vi "AnalogAcquisition.vi"() -> ()   [LabVIEW 2017]
uses:
  <vilib>/DAQmx/create/channels.llb/DAQmx Create Channel (AI-Voltage-Basic).vi
  <vilib>/DAQmx/read.llb/DAQmx Read (Analog 1D DBL NChan 1Samp).vi
  <vilib>/DAQmx/configure/timing.llb/DAQmx Timing (Sample Clock).vi
  <vilib>/DAQmx/create/channels.llb/DAQmx Create Channel (AI-Current-Basic).vi
panel:
  out "KnobDistance 1.4":dbl[](array[numeric])
  out "KnobDistance 2.4":dbl[](array[numeric])
  out "KnobDistance 2.3":dbl[](array[numeric])
  out "KnobDistance 2.2":dbl[](array[numeric])
  out "KnobDistance 2.1":dbl[](array[numeric])
  out "KnobDistance 1.3":dbl[](array[numeric])
  out "KnobDistance 1.2":dbl[](array[numeric])
  out "KnobDistance 1.1":dbl[](array[numeric])
  out "BufferWDWArray 2.3":T1
  out "BufferWDWArray 2.4":T1
  out "BufferWDWArray 2.1":T1
  out "BufferWDWArray 2.2":T1
  out "BufferWDWArray 1.3":T1
  out "BufferWDWArray 1.4":T1
  out "BufferWDWArray 1.1":T1
  out "BufferWDWArray 1.2":T1
  out "WDW Judge 2":bool
  out "WDW Judge":bool
  out "SamplingRate":i32
  in  "stop":bool
  out "WDW_Read 2":bool
  out "RL_Read 2":bool
  out "FL_Read 2":bool
  out "RR_Read 2":bool
  out "FR_Read 2":bool
  out "DL_Read 2":bool
  out "RL_Read 1":bool
  out "FL_Read 1":bool
  out "RR_Read 1":bool
  out "FR_Read 1":bool
  out "DL_Read 1":bool
  out "WDW_Read 1":bool
  out "Flash":bool
  out "BufferRLArray 2.3":T2
  out "BufferRLArray 2.4":T2
  out "BufferFLArray 2.3":T2
  out "BufferFLArray 2.4":T2
  out "BufferRRArray 2.3":T2
  out "BufferRRArray 2.4":T2
  out "BufferFRArray 2.3":T2
  out "BufferFRArray 2.4":T2
  out "BufferDLArray 2.4":T2
  out "BufferDLArray 2.3":T2
  out "BufferRLArray 1.3":T2
  out "BufferRLArray 1.4":T2
  out "BufferFLArray 1.3":T2
  out "BufferFLArray 1.4":T2
  out "BufferRRArray 1.3":T2
  out "BufferRRArray 1.4":T2
  out "BufferFRArray 1.3":T2
  out "BufferFRArray 1.4":T2
  out "BufferDLArray 1.4":T2
  out "BufferDLArray 1.3":T2
  out "BufferRLArray 2.1":T2
  out "BufferRLArray 2.2":T2
  out "BufferFLArray 2.1":T2
  out "BufferFLArray 2.2":T2
  out "BufferRRArray 2.1":T2
  out "BufferRRArray 2.2":T2
  out "BufferFRArray 2.1":T2
  out "BufferFRArray 2.2":T2
  out "BufferDLArray 2.2":T2
  out "BufferDLArray 2.1":T2
  out "BufferRLArray 1.1":T2
  out "BufferRLArray 1.2":T2
  out "BufferFLArray 1.1":T2
  out "BufferFLArray 1.2":T2
  out "BufferRRArray 1.1":T2
  out "BufferRRArray 1.2":T2
  out "BufferFRArray 1.1":T2
  out "BufferFRArray 1.2":T2
  out "BufferDLArray 1.2":T2
  out "BufferDLArray 1.1":T2
  out "RL Judge 2":bool
  out "FL Judge 2":bool
  out "RR Judge 2":bool
  out "FR Judge 2":bool
  out "DoorLock Judge 2":bool
  out "RL Judge":bool
  out "FL Judge":bool
  out "RR Judge":bool
  out "FR Judge":bool
  out "DoorLock Judge":bool
  # "ANALOG ACQUISITION"
  # "ITEM"
  # "LANE 1"
  # "LANE 2"
  # "WDW LOCK /UNLOCK"
  # "DOOR LOCK /UNLOCK"
  # "FR Up/DOWN"
  # "RR Up/DOWN"
  # "FL Up/DOWN"
  # "RL Up/DOWN"
  # "/Sec."
  # "SAMPLING RATE"
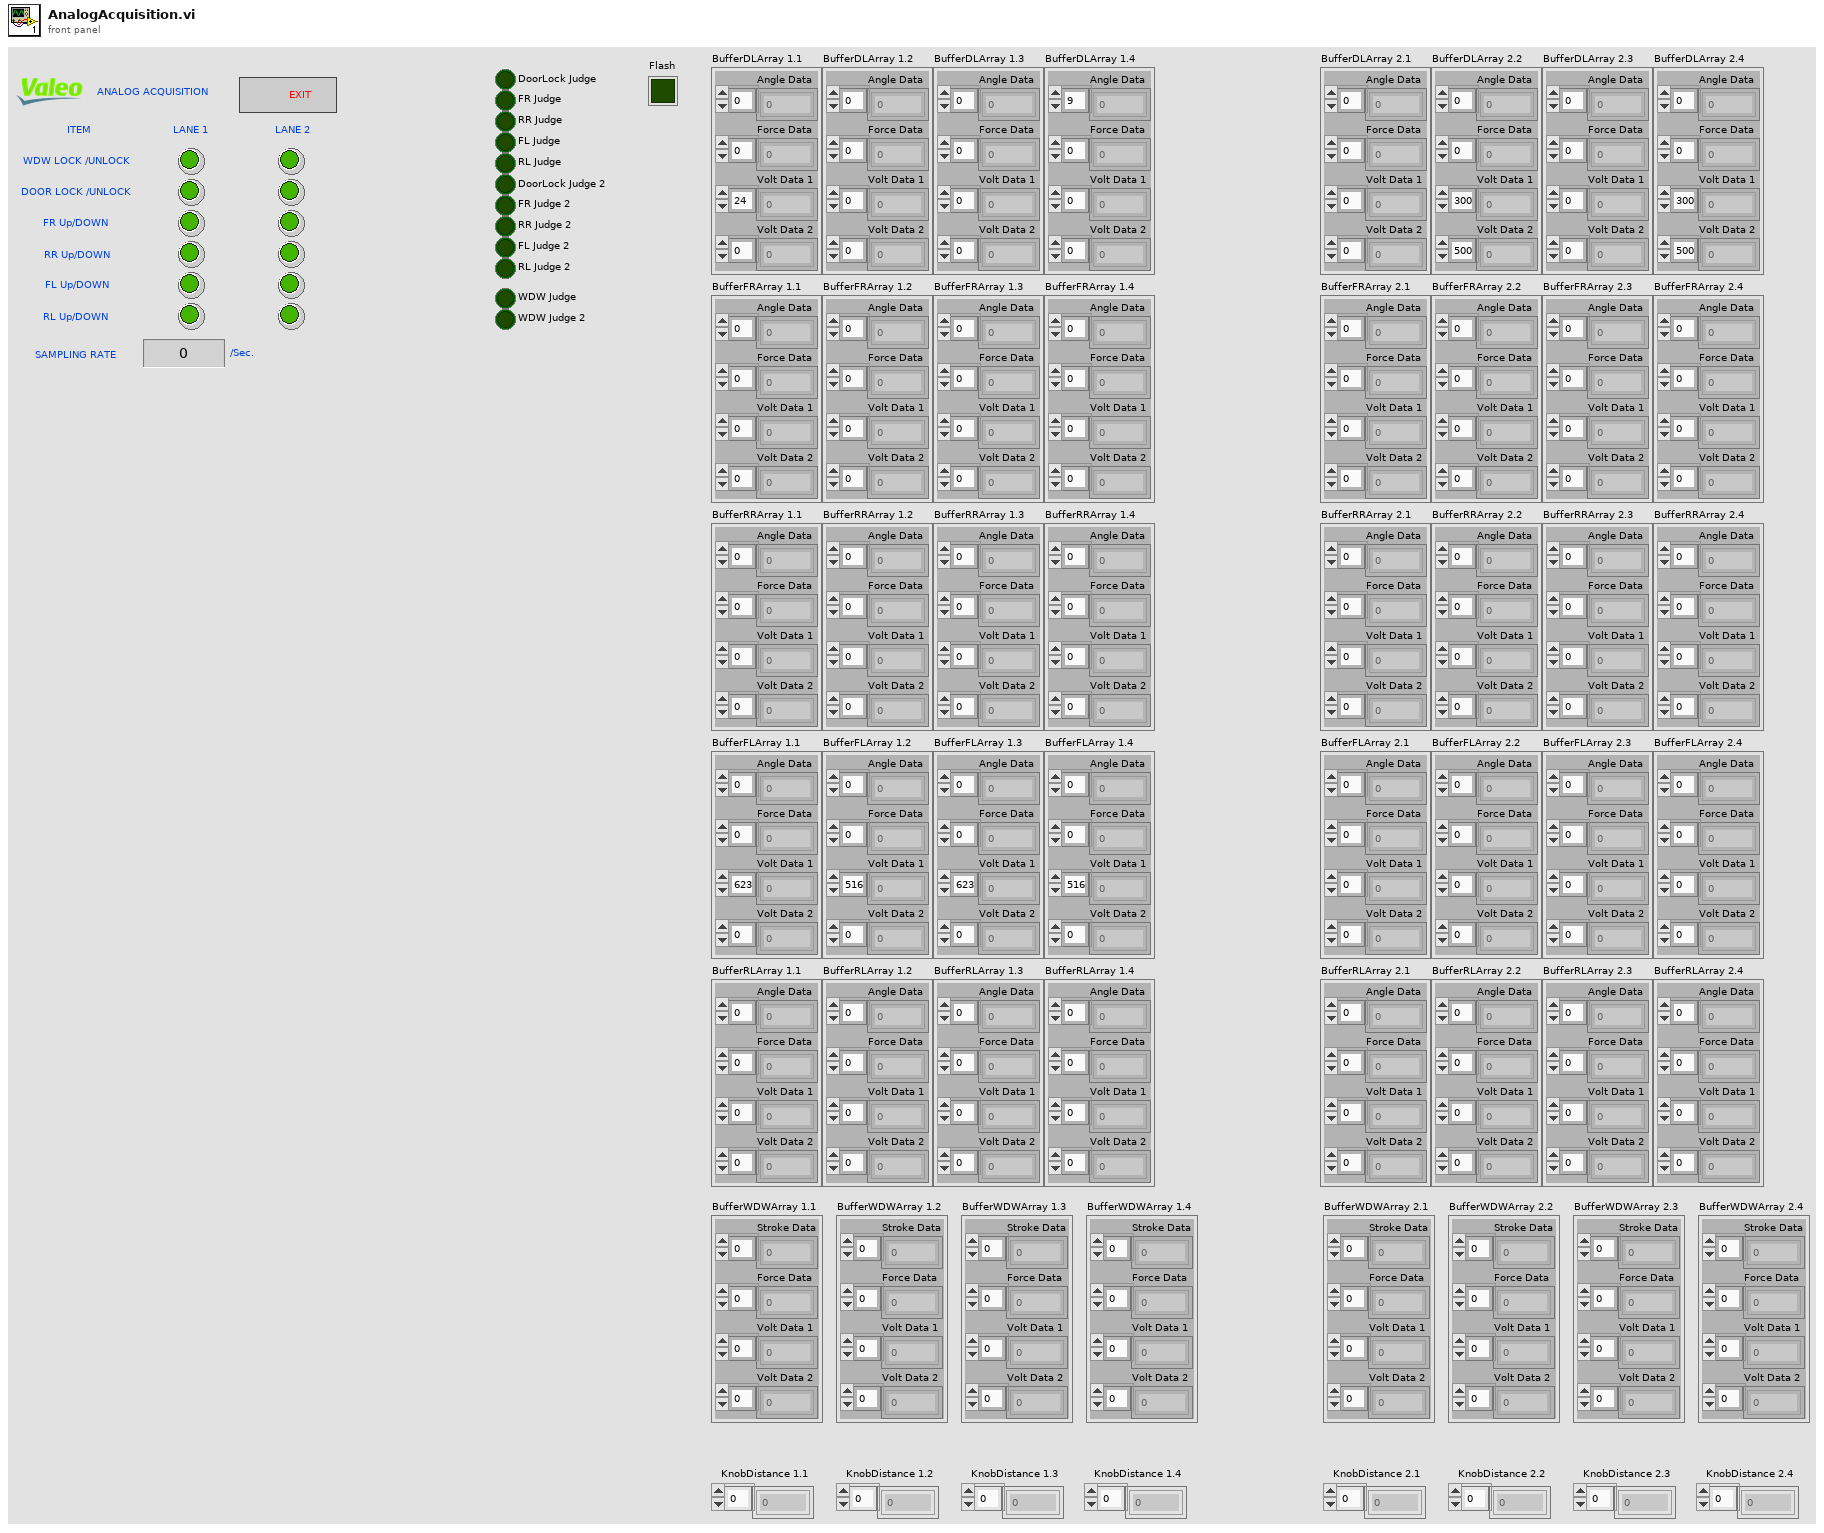
[diagram p1: front panel]
types:
  T1 = cluster{"Stroke Data":dbl[], "Force Data":dbl[], "Volt Data 1":dbl[], "Volt Data 2":dbl[]}
  T2 = cluster{"Angle Data":dbl[], "Force Data":dbl[], "Volt Data 1":dbl[], "Volt Data 2":dbl[]}
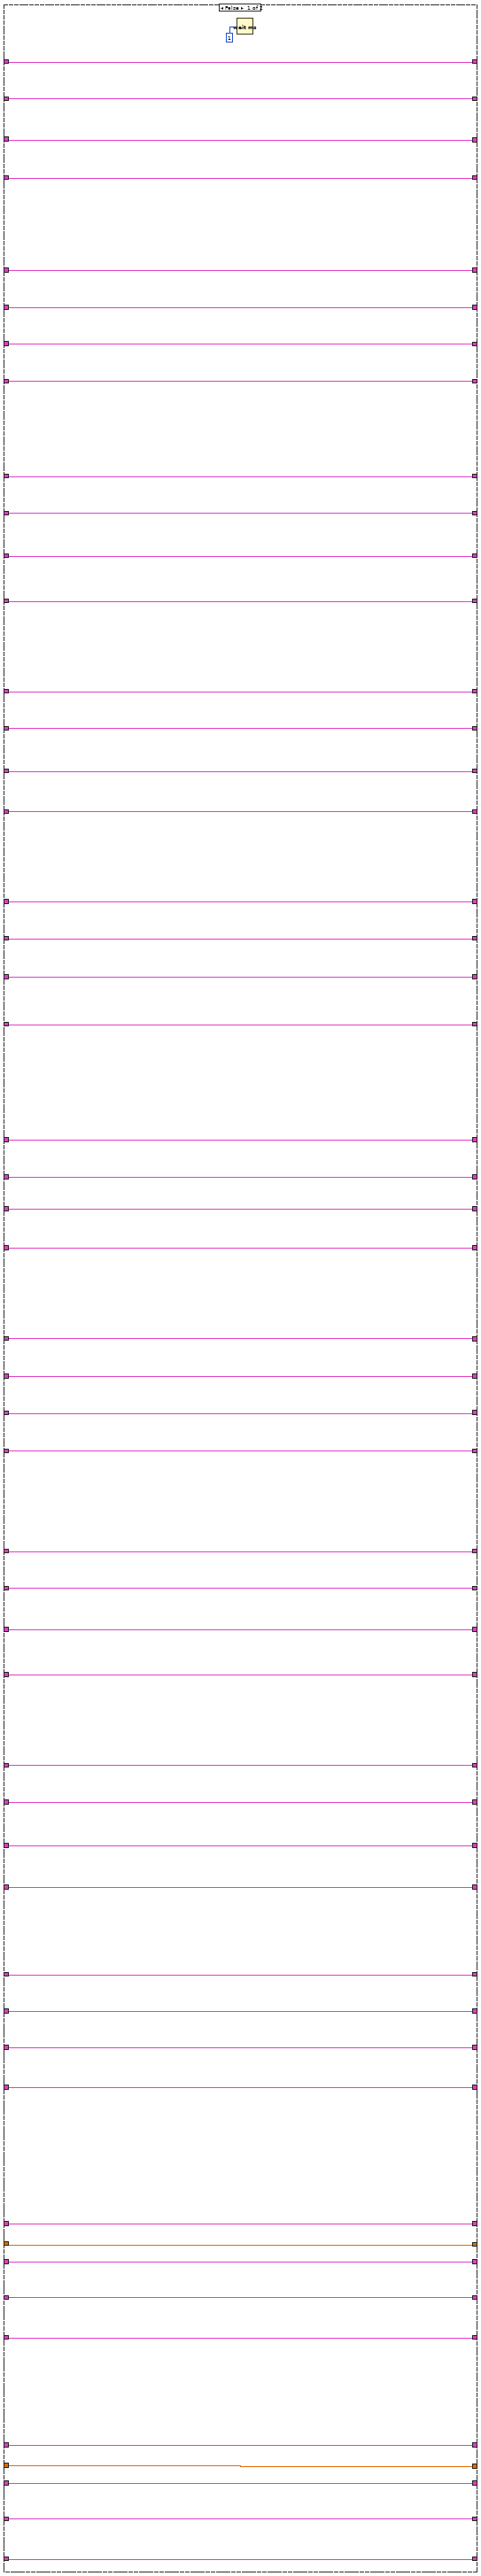
[diagram p5: hidden frame]
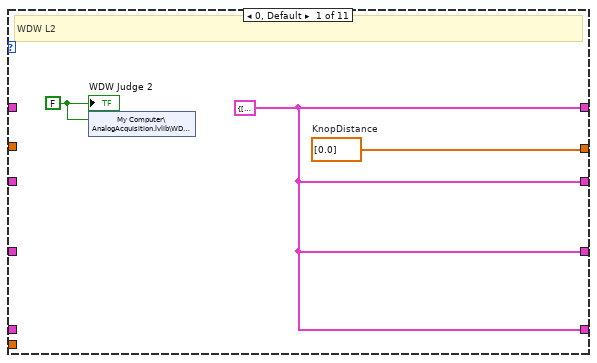
[diagram p6: hidden frame]
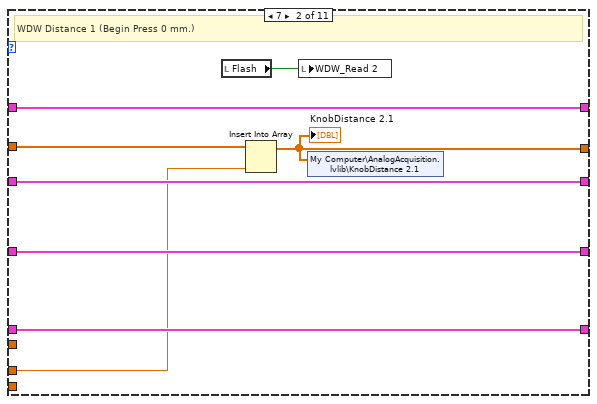
[diagram p7: hidden frame]
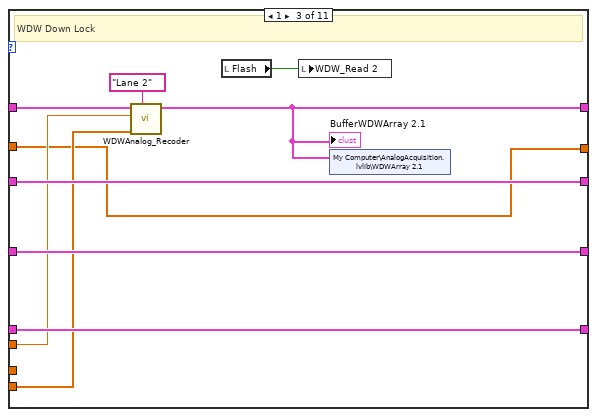
[diagram p8: hidden frame]
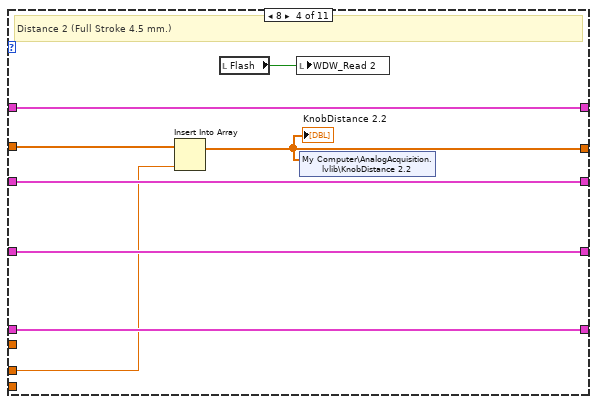
[diagram p9: hidden frame]
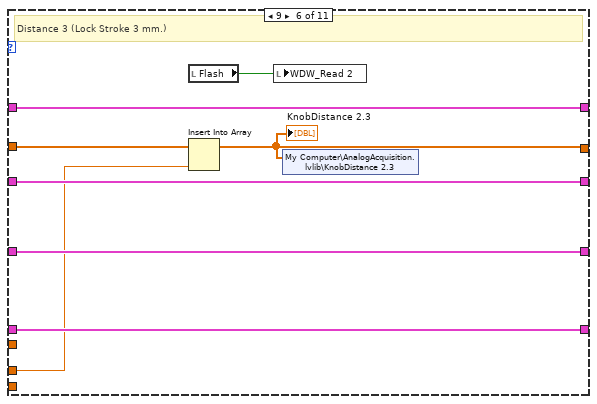
[diagram p10: hidden frame]
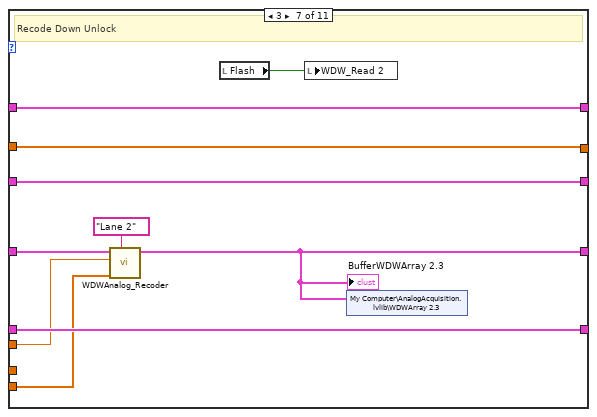
[diagram p11: hidden frame]
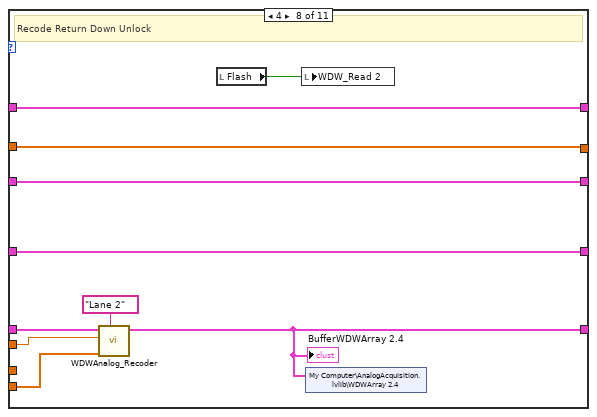
[diagram p12: hidden frame]
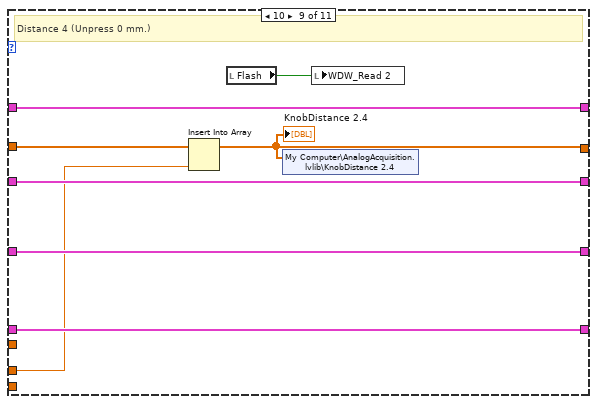
[diagram p13: hidden frame]
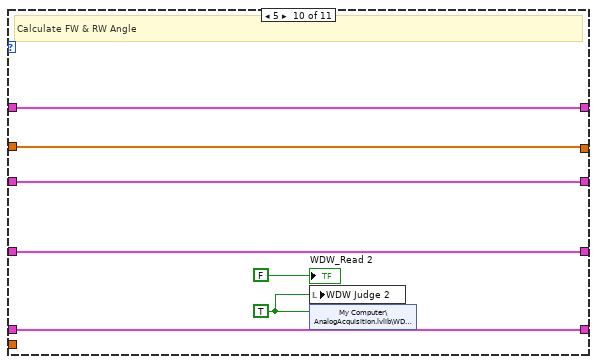
[diagram p14: hidden frame]
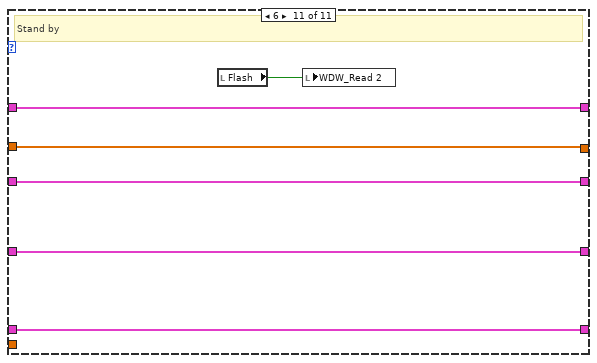
[diagram p15: hidden frame]
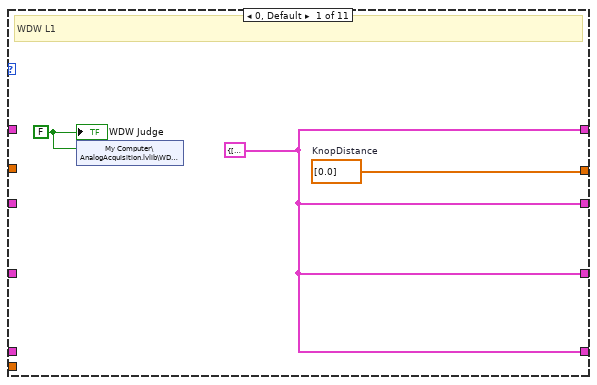
[diagram p16: hidden frame]
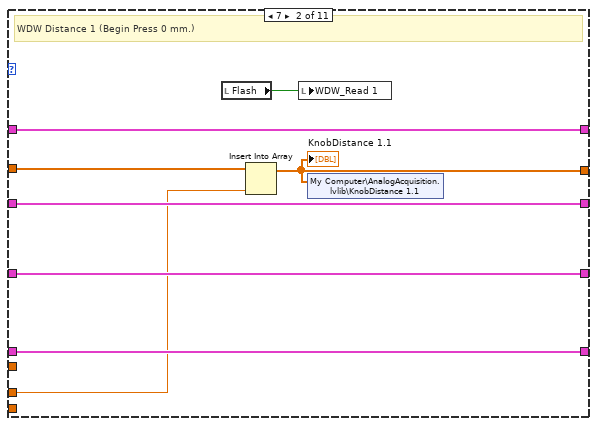
[diagram p17: hidden frame]
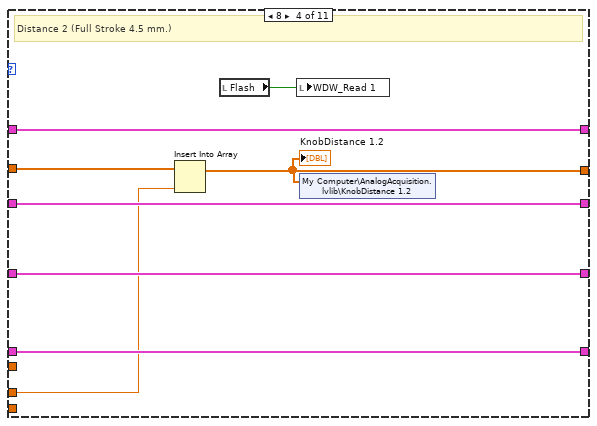
[diagram p18: hidden frame]
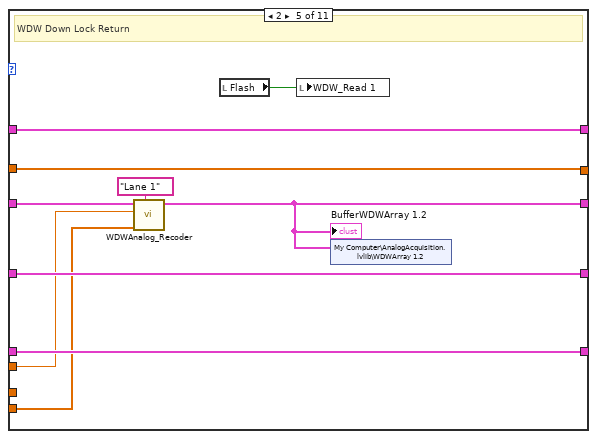
[diagram p19: hidden frame]
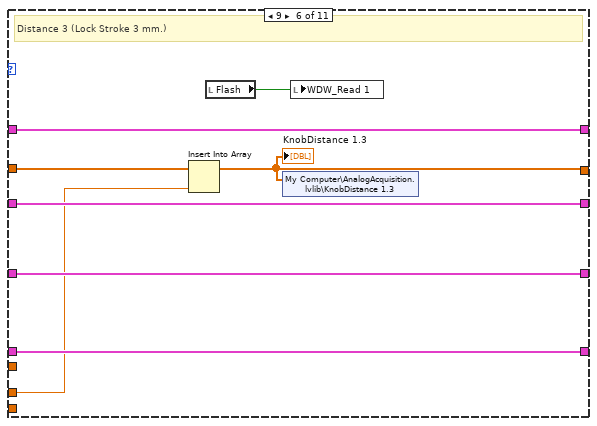
[diagram p20: hidden frame]
diagram:
  w7 = dbl[] [0.0]  # KnopDistance
  w5 = T2 {"Angle Data"=[0.0], "Force Data"=[0.0], "Volt Data 1"=[0.0], "Volt Data 2"=[0.0]} ("Analog Array Out")
  n1 = flat-sequence {
    frame #0 {
      n2 = control-ref of="This VI"() -> (w12:refnum<vi>)
      n3 = invoke class="VI" method="Default Vals.Reinit All"(reference=w12) -> ()  [unwired: 2 in, 3 out]
    }
    frame #1 {
      n4 = Wait (ms)(milliseconds to wait=u32 100) -> ()  [unwired: 1 out]
    }
    frame #2 {
      w14 = FALSE ("DoorLock Judge")
      n5 = local write "DoorLock Judge 2"(w14) -> ()
      n6 = local write "DoorLock Judge"(w14) -> ()
      n7 = shared-variable "My Computer\\AnalogAcquisition.lvlib\\WDW_1_OK"(w14) -> ()  [unwired: 1 in, 1 out]
      n8 = shared-variable "My Computer\\AnalogAcquisition.lvlib\\WDW_2_OK"(w14) -> ()  [unwired: 1 in, 1 out]
      n9 = shared-variable "My Computer\\AnalogAcquisition.lvlib\\DL_1_OK"(w14) -> ()  [unwired: 1 in, 1 out]
      n10 = shared-variable "My Computer\\AnalogAcquisition.lvlib\\DL_2_OK"(w14) -> ()  [unwired: 1 in, 1 out]
      n11 = shared-variable "My Computer\\AnalogAcquisition.lvlib\\RR_1_OK"(w14) -> ()  [unwired: 1 in, 1 out]
      n12 = shared-variable "My Computer\\AnalogAcquisition.lvlib\\RR_2_OK"(w14) -> ()  [unwired: 1 in, 1 out]
      n13 = shared-variable "My Computer\\AnalogAcquisition.lvlib\\FR_1_OK"(w14) -> ()  [unwired: 1 in, 1 out]
      n14 = shared-variable "My Computer\\AnalogAcquisition.lvlib\\FR_2_OK"(w14) -> ()  [unwired: 1 in, 1 out]
      n15 = shared-variable "My Computer\\AnalogAcquisition.lvlib\\RL_1_OK"(w14) -> ()  [unwired: 1 in, 1 out]
      n16 = shared-variable "My Computer\\AnalogAcquisition.lvlib\\RL_2_OK"(w14) -> ()  [unwired: 1 in, 1 out]
      n17 = shared-variable "My Computer\\AnalogAcquisition.lvlib\\FL_1_OK"(w14) -> ()  [unwired: 1 in, 1 out]
      n18 = shared-variable "My Computer\\AnalogAcquisition.lvlib\\FL_2_OK"(w14) -> ()  [unwired: 1 in, 1 out]
      n19 = local write "RR Judge 2"(w14) -> ()
      n20 = local write "FR Judge 2"(w14) -> ()
      n21 = local write "RL Judge 2"(w14) -> ()
      n22 = local write "FL Judge 2"(w14) -> ()
      n23 = local write "RR Judge"(w14) -> ()
      n24 = local write "FR Judge"(w14) -> ()
      n25 = local write "RL Judge"(w14) -> ()
      n26 = local write "FL Judge"(w14) -> ()
    }
  }
  n27 = disable-structure shown="Enabled" {
    disable-tunnel: [w23 _] -> w11
    disable-tunnel: [w22 _] -> w10
    frame Enabled {
      w17 = 10123 items=["Finite Samples"=10178, "Continuous Samples"=10123, "Hardware Timed Single Point"=12522] ("sample mode")
      n28 = call-poly <vilib>:"DAQmx Create Virtual Channel.vi"("physical channels"=tag "cDAQ9189-1D361EBMod1/ai0:7, cDAQ9189-1D361EBMod2/ai0:7, cDAQ9189-1D361EBMod3/ai0:7, cDAQ9189-1D361EBMod4/ai0:7, cDAQ9189-1D361EBMod5/ai0:7", "error in"=errorcluster {"status"=FALSE, "code"=0, "source"=""} ("error constant")) -> ("task out"=w21:refnum<k21>, "error out"=w20:errorcluster)  [unwired: 12 in]
      n29 = call-poly <vilib>:"DAQmx Timing.vi"("task/channels in"=w21, "sample mode"=w17, "samples per channel"=650, "rate"=650.0, "error in"=w20) -> ("task out"=w18:refnum<k21>, "error out"=w19:errorcluster)  [unwired: 9 in]
      n30 = call <vilib>:"DAQmx Start Task.vi"("task/channels in"=w18, "error in"=w19) -> ("task out"=w23:refnum<k21>, "error out"=w22:errorcluster)  [unwired: 12 in]
    }
    frame Disabled {
    }
  }
  n31 = disable-structure shown="Enabled" {
    disable-tunnel: [w27 _] -> w4
    disable-tunnel: [w26 _] -> w3
    frame Enabled {
      w29 = 10123 items=["Finite Samples"=10178, "Continuous Samples"=10123, "Hardware Timed Single Point"=12522] ("sample mode")
      n32 = call-poly <vilib>:"DAQmx Create Virtual Channel.vi"("physical channels"=tag "cDAQ9189-1D361EBMod6/ai0:1", "error in"=errorcluster {"status"=FALSE, "code"=0, "source"=""} ("error constant")) -> ("task out"=w34:refnum<k21>, "error out"=w33:errorcluster)  [unwired: 12 in]
      n33 = call-poly <vilib>:"DAQmx Timing.vi"("task/channels in"=w34, "sample mode"=w29, "samples per channel"=650, "rate"=650.0, "error in"=w33) -> ("task out"=w31:refnum<k21>, "error out"=w32:errorcluster)  [unwired: 9 in]
      n34 = call <vilib>:"DAQmx Start Task.vi"("task/channels in"=w31, "error in"=w32) -> ("task out"=w27:refnum<k21>, "error out"=w26:errorcluster)  [unwired: 12 in]
    }
    frame Disabled {
    }
  }
  n35 = while {
    shift-right: [w143] -> w9
    shift-left: w11 -> [w144]
    shift-right: [w142] -> w8
    shift-left: w10 -> [w141]
    shift-right: [w165] -> _
    shift-left: w5 -> [w167]
    shift-right: [w164] -> _
    shift-left: w5 -> [w166]
    shift-right: [w161] -> _
    shift-left: w5 -> [w163]
    shift-right: [w160] -> _
    shift-left: w5 -> [w162]
    shift-right: [w138] -> _
    shift-left: w5 -> [w159]
    shift-right: [w137] -> _
    shift-left: w5 -> [w158]
    shift-right: [w136] -> _
    shift-left: w5 -> [w156]
    shift-right: [w135] -> _
    shift-left: w5 -> [w157]
    shift-right: [w134] -> _
    shift-left: w5 -> [w155]
    shift-right: [w133] -> _
    shift-left: w5 -> [w154]
    shift-right: [w132] -> _
    shift-left: w5 -> [w145]
    shift-right: [w131] -> _
    shift-left: w5 -> [w146]
    shift-right: [w130] -> _
    shift-left: w5 -> [w140]
    shift-right: [w129] -> _
    shift-left: w5 -> [w147]
    shift-right: [w128] -> _
    shift-left: w5 -> [w148]
    shift-right: [w127] -> _
    shift-left: w5 -> [w149]
    shift-right: [w126] -> _
    shift-left: w5 -> [w151]
    shift-right: [w125] -> _
    shift-left: w5 -> [w150]
    shift-right: [w124] -> _
    shift-left: w5 -> [w152]
    shift-right: [w123] -> _
    shift-left: w5 -> [w153]
    shift-right: [w121] -> _
    shift-left: w5 -> [w122]
    shift-right: [w120] -> _
    shift-left: w5 -> [w119]
    shift-right: [w118] -> _
    shift-left: w5 -> [w117]
    shift-right: [w116] -> _
    shift-left: w5 -> [w115]
    shift-right: [w114] -> _
    shift-left: w5 -> [w113]
    shift-right: [w112] -> _
    shift-left: w5 -> [w111]
    shift-right: [w109] -> _
    shift-left: w5 -> [w110]
    shift-right: [w108] -> _
    shift-left: w5 -> [w107]
    shift-right: [w106] -> _
    shift-left: w5 -> [w105]
    shift-right: [w104] -> _
    shift-left: w5 -> [w103]
    shift-right: [w102] -> _
    shift-left: w5 -> [w101]
    shift-right: [w100] -> _
    shift-left: w5 -> [w99]
    shift-right: [w97] -> _
    shift-left: w5 -> [w98]
    shift-right: [w96] -> _
    shift-left: w5 -> [w95]
    shift-right: [w94] -> _
    shift-left: w5 -> [w93]
    shift-right: [w92] -> _
    shift-left: w5 -> [w91]
    shift-right: [w90] -> _
    shift-left: w5 -> [w89]
    shift-right: [w88] -> _
    shift-left: w5 -> [w87]
    shift-right: [w84] -> _
    shift-left: w5 -> [w86]
    shift-right: [w83] -> _
    shift-left: w5 -> [w85]
    shift-right: [w65] -> _
    shift-left: w5 -> [w64]
    shift-right: [w59] -> _
    shift-left: w5 -> [w58]
    shift-right: [w62] -> _
    shift-left: w5 -> [w60]
    shift-right: [w63] -> _
    shift-left: w5 -> [w61]
    shift-right: [w50] -> _
    shift-left: w5 -> [w51]
    shift-right: [w56] -> _
    shift-left: w5 -> [w57]
    shift-right: [w53] -> _
    shift-left: w5 -> [w55]
    shift-right: [w52] -> _
    shift-left: w5 -> [w54]
    shift-right: [w48] -> _
    shift-left: w7 -> [w49]
    shift-right: [w47] -> _
    shift-left: w7 -> [w46]
    tunnel: [w45] -> w6
    tunnel: w4 -> [w42]
    tunnel: w3 -> [w41]
    tunnel: [w40] -> w2
    tunnel: [w39] -> w1
    i -> [w70]
    stop <- w45 stop-if-true
    # "Read Analog Input"
    n36 = shared-variable "My Computer\\SerialStepForce.lvlib\\Serial OK"() -> (w66:bool)  [unwired: 1 in, 1 out]
    n37 = disable-structure shown="Enabled" {
      disable-tunnel: w144 -> [w1007 _]
      disable-tunnel: [w1006 _] -> w143
      disable-tunnel: [w1005 _] -> w142
      disable-tunnel: w141 -> [w1004 _]
      disable-tunnel: [w1003 _] -> w139
      frame Enabled {
        n38 = call-poly <vilib>:"DAQmx Read.vi"("task/channels in"=w1007, "error in"=w1004) -> ("task out"=w1006:refnum<k21>, "data"=w1003:dbl[], "error out"=w1005:errorcluster)  [unwired: 11 in]
      }
      frame Disabled {
      }
    }
    n39 = local read "DL_Read 1"() -> (w73:bool)
    n40 = local read "FR_Read 1"() -> (w74:bool)
    n41 = local read "RR_Read 1"() -> (w75:bool)
    n42 = local read "FL_Read 1"() -> (w76:bool)
    n43 = local read "RL_Read 1"() -> (w77:bool)
    n44 = local read "DL_Read 2"() -> (w78:bool)
    n45 = local read "FR_Read 2"() -> (w79:bool)
    n46 = local read "RR_Read 2"() -> (w72:bool)
    n47 = local read "FL_Read 2"() -> (w80:bool)
    n48 = local read "RL_Read 2"() -> (w71:bool)
    n49 = local read "WDW_Read 1"() -> (w44:bool)
    n50 = local read "WDW_Read 2"() -> (w43:bool)
    n51 = call-poly <vilib>:"DAQmx Read.vi"("task/channels in"=w42, "error in"=w41) -> ("task out"=w40:refnum<k21>, "data"=w38:dbl[], "error out"=w39:errorcluster)  [unwired: 11 in]
    n52 = Absolute Value(x=w38) -> (abs(x)=w37:dbl[])
    n53 = case shown="True" w66 {
      tunnel: w167 -> [w218 w336]
      tunnel: w166 -> [w217 w335]
      tunnel: [w218 w334] -> w165
      tunnel: [w217 w333] -> w164
      tunnel: w163 -> [w212 w332]
      tunnel: w162 -> [w211 w331]
      tunnel: [w212 w330] -> w161
      tunnel: [w211 w329] -> w160
      tunnel: w159 -> [w210 w328]
      tunnel: w158 -> [w209 w327]
      tunnel: w157 -> [w205 w326]
      tunnel: w156 -> [w206 w325]
      tunnel: w155 -> [w202 w324]
      tunnel: w154 -> [w201 w323]
      tunnel: w153 -> [w181 w322]
      tunnel: w152 -> [w182 w321]
      tunnel: w151 -> [w186 w320]
      tunnel: w150 -> [w185 w319]
      tunnel: w149 -> [w189 w318]
      tunnel: w148 -> [w190 w317]
      tunnel: w147 -> [w193 w316]
      tunnel: w146 -> [w197 w315]
      tunnel: w145 -> [w198 w314]
      tunnel: w140 -> [w194 w313]
      tunnel: w139 -> [_ w223]
      tunnel: [w210 w312] -> w138
      tunnel: [w209 w311] -> w137
      tunnel: [w206 w310] -> w136
      tunnel: [w205 w309] -> w135
      tunnel: [w202 w308] -> w134
      tunnel: [w201 w307] -> w133
      tunnel: [w198 w306] -> w132
      tunnel: [w197 w305] -> w131
      tunnel: [w194 w304] -> w130
      tunnel: [w193 w303] -> w129
      tunnel: [w190 w302] -> w128
      tunnel: [w189 w301] -> w127
      tunnel: [w186 w300] -> w126
      tunnel: [w185 w299] -> w125
      tunnel: [w182 w298] -> w124
      tunnel: [w181 w297] -> w123
      tunnel: w122 -> [w216 w286]
      tunnel: [w216 w285] -> w121
      tunnel: [w215 w284] -> w120
      tunnel: w119 -> [w215 w283]
      tunnel: [w214 w282] -> w118
      tunnel: w117 -> [w214 w281]
      tunnel: [w213 w280] -> w116
      tunnel: w115 -> [w213 w279]
      tunnel: [w208 w278] -> w114
      tunnel: w113 -> [w208 w277]
      tunnel: [w207 w276] -> w112
      tunnel: w111 -> [w207 w275]
      tunnel: w110 -> [w204 w274]
      tunnel: [w204 w273] -> w109
      tunnel: [w203 w272] -> w108
      tunnel: w107 -> [w203 w271]
      tunnel: [w200 w270] -> w106
      tunnel: w105 -> [w200 w269]
      tunnel: [w199 w268] -> w104
      tunnel: w103 -> [w199 w267]
      tunnel: [w196 w266] -> w102
      tunnel: w101 -> [w196 w265]
      tunnel: [w195 w264] -> w100
      tunnel: w99 -> [w195 w263]
      tunnel: w98 -> [w192 w262]
      tunnel: [w192 w261] -> w97
      tunnel: [w191 w260] -> w96
      tunnel: w95 -> [w191 w259]
      tunnel: [w188 w258] -> w94
      tunnel: w93 -> [w188 w257]
      tunnel: [w187 w256] -> w92
      tunnel: w91 -> [w187 w255]
      tunnel: [w184 w254] -> w90
      tunnel: w89 -> [w184 w253]
      tunnel: [w183 w252] -> w88
      tunnel: w87 -> [w183 w251]
      tunnel: w86 -> [w180 w250]
      tunnel: w85 -> [w179 w249]
      tunnel: [w180 w248] -> w84
      tunnel: [w179 w247] -> w83
      tunnel: [w177 w245] -> w65
      tunnel: w64 -> [w177 w244]
      tunnel: w58 -> [w174 w242]
      tunnel: [w174 w241] -> w59
      tunnel: w60 -> [w175 w239]
      tunnel: w61 -> [w176 w237]
      tunnel: [w175 w240] -> w62
      tunnel: [w176 w238] -> w63
      tunnel: [w173 w230] -> w50
      tunnel: w51 -> [w173 w233]
      tunnel: w57 -> [w172 w229]
      tunnel: [w172 w228] -> w56
      tunnel: w55 -> [w171 w227]
      tunnel: w54 -> [w170 w224]
      tunnel: [w171 w226] -> w53
      tunnel: [w170 w225] -> w52
      tunnel: w49 -> [w169 w235]
      tunnel: [w169 w236] -> w48
      tunnel: [w168 w231] -> w47
      tunnel: w46 -> [w168 w232]
      tunnel: w37 -> [_ w220]
      frame False {
        n54 = Wait (ms)(milliseconds to wait=u32 1) -> ()  [unwired: 1 out]
      }
      frame True {
        # "WDW Lane 2"
        # "WDW Lane 1"
        # "Lane 1"
        # "Lane 2"
        n55 = shared-variable "My Computer\\SerialStepForce.lvlib\\Step Force"() -> (w246:u8[])  [unwired: 1 in, 1 out]
        n56 = Index Array(array=w220, index #1=0 ("index")) -> (element #1=w221:dbl, element #2=w219:dbl)  [unwired: 1 in]
        n57 = Index Array(array=w246) -> (element #1=w296:u8, element #2=w295:u8, element #3=w294:u8, element #4=w293:u8, element #5=w292:u8, element #6=w291:u8, element #7=w290:u8, element #8=w289:u8, element #9=w288:u8, element #10=w287:u8, element #11=w243:u8, element #12=w234:u8)  [unwired: 12 in]
        n58 = case shown="1" w243 {
          tunnel: [w426 w431 w437 w452 w462 w470 w480 w490 w498 w504 w511] -> w245
          tunnel: w244 -> [_ w431 w441 w452 w462 w470 w480 w490 w498 w504 w511]
          tunnel: w242 -> [_ w434 w444 w449 w458 w469 w479 w489 w497 w501 w510]
          tunnel: [w426 w434 w444 w449 w455 w469 w479 w489 w497 w501 w510] -> w241
          tunnel: [w426 w433 w443 w451 w461 w468 w473 w488 w496 w503 w509] -> w240
          tunnel: w239 -> [_ w433 w443 w451 w461 w468 w476 w488 w496 w503 w509]
          tunnel: [w426 w432 w442 w450 w460 w467 w478 w483 w495 w502 w508] -> w238
          tunnel: w237 -> [_ w432 w442 w450 w460 w467 w478 w486 w495 w502 w508]
          tunnel: w221 -> [_ _ w439 _ w457 _ w475 w485 _ _ _]
          tunnel: w219 -> [_ w429 _ w447 _ w465 _ _ w493 _ _]
          tunnel: w223 -> [_ _ w438 _ w456 _ w474 w484 _ _ _]
          tunnel: w235 -> [_ w430 w436 w448 w454 w466 w472 w482 w494 w500 w507]
          tunnel: [w425 w428 w436 w446 w454 w464 w472 w482 w492 w500 w507] -> w236
          frame 0, Default {
            w425 = dbl[] [0.0]  # KnopDistance
            w427 = FALSE ("RL Judge")
            w426 = T1 {"Stroke Data"=[], "Force Data"=[], "Volt Data 1"=[], "Volt Data 2"=[]} ("Analog Array Out")
            # "WDW L1"
            n59 = shared-variable "My Computer\\AnalogAcquisition.lvlib\\WDW_1_OK"(w427) -> ()  [unwired: 1 in, 1 out]
            "WDW Judge" <- w427
          }
          frame 7 {
            # "WDW Distance 1 (Begin Press 0 mm.)"
            n60 = local read "Flash"() -> (w435:bool)
            n61 = Insert Into Array(array=w430, new element=w429) -> (w428:dbl[])  [unwired: 1 in]
            "KnobDistance 1.1" <- w428
            n62 = local write "WDW_Read 1"(w435) -> ()
            n63 = shared-variable "My Computer\\AnalogAcquisition.lvlib\\KnobDistance 1.1"(w428) -> ()  [unwired: 1 in, 1 out]
          }
          frame 1 {
            # "WDW Down Lock"
            n64 = call "WDWAnalog_Recoder.vi"("Lane Number"="Lane 1", "Analog Data In"=w438, "ForceData"=w439, "Analog Array In"=w441) -> ("Analog Array Out"=w437:T1)  [unwired: 7 in]
            "BufferWDWArray 1.1" <- w437
            n65 = local read "Flash"() -> (w445:bool)
            n66 = local write "WDW_Read 1"(w445) -> ()
            n67 = shared-variable "My Computer\\AnalogAcquisition.lvlib\\WDWArray 1.1"(w437) -> ()  [unwired: 1 in, 1 out]
          }
          frame 8 {
            # "Distance 2 (Full Stroke 4.5 mm.)"
            n68 = Insert Into Array(array=w448, new element=w447) -> (w446:dbl[])  [unwired: 1 in]
            "KnobDistance 1.2" <- w446
            n69 = local read "Flash"() -> (w453:bool)
            n70 = local write "WDW_Read 1"(w453) -> ()
            n71 = shared-variable "My Computer\\AnalogAcquisition.lvlib\\KnobDistance 1.2"(w446) -> ()  [unwired: 1 in, 1 out]
          }
          frame 2 {
            # "WDW Down Lock Return"
            n72 = call "WDWAnalog_Recoder.vi"("Lane Number"="Lane 1", "Analog Data In"=w456, "ForceData"=w457, "Analog Array In"=w458) -> ("Analog Array Out"=w455:T1)  [unwired: 7 in]
            "BufferWDWArray 1.2" <- w455
            n73 = local read "Flash"() -> (w463:bool)
            n74 = local write "WDW_Read 1"(w463) -> ()
            n75 = shared-variable "My Computer\\AnalogAcquisition.lvlib\\WDWArray 1.2"(w455) -> ()  [unwired: 1 in, 1 out]
          }
          frame 9 {
            # "Distance 3 (Lock Stroke 3 mm.)"
            n76 = Insert Into Array(array=w466, new element=w465) -> (w464:dbl[])  [unwired: 1 in]
            "KnobDistance 1.3" <- w464
            n77 = local read "Flash"() -> (w471:bool)
            n78 = shared-variable "My Computer\\AnalogAcquisition.lvlib\\KnobDistance 1.3"(w464) -> ()  [unwired: 1 in, 1 out]
            n79 = local write "WDW_Read 1"(w471) -> ()
          }
          frame 3 {
            # "Recode Down Unlock"
            n80 = call "WDWAnalog_Recoder.vi"("Lane Number"="Lane 1", "Analog Data In"=w474, "ForceData"=w475, "Analog Array In"=w476) -> ("Analog Array Out"=w473:T1)  [unwired: 7 in]
            "BufferWDWArray 1.3" <- w473
            n81 = local read "Flash"() -> (w481:bool)
            n82 = local write "WDW_Read 1"(w481) -> ()
            n83 = shared-variable "My Computer\\AnalogAcquisition.lvlib\\WDWArray 1.3"(w473) -> ()  [unwired: 1 in, 1 out]
          }
          frame 4 {
            # "Recode Return Down Unlock"
            n84 = call "WDWAnalog_Recoder.vi"("Lane Number"="Lane 1", "Analog Data In"=w484, "ForceData"=w485, "Analog Array In"=w486) -> ("Analog Array Out"=w483:T1)  [unwired: 7 in]
            "BufferWDWArray 1.4" <- w483
            n85 = local read "Flash"() -> (w491:bool)
            n86 = shared-variable "My Computer\\AnalogAcquisition.lvlib\\WDWArray 1.4"(w483) -> ()  [unwired: 1 in, 1 out]
            n87 = local write "WDW_Read 1"(w491) -> ()
          }
          frame 10 {
            # "Distance 4 (Unpress 0 mm.)"
            n88 = Insert Into Array(array=w494, new element=w493) -> (w492:dbl[])  [unwired: 1 in]
            "KnobDistance 1.4" <- w492
            n89 = local read "Flash"() -> (w499:bool)
            n90 = shared-variable "My Computer\\AnalogAcquisition.lvlib\\KnobDistance 1.4"(w492) -> ()  [unwired: 1 in, 1 out]
            n91 = local write "WDW_Read 1"(w499) -> ()
          }
          frame 5 {
            w506 = TRUE ("RL Judge 2")
            # "Calculate FW & RW Angle"
            n92 = local write "WDW Judge"(w506) -> ()
            n93 = shared-variable "My Computer\\AnalogAcquisition.lvlib\\WDW_1_OK"(w506) -> ()  [unwired: 1 in, 1 out]
            "WDW_Read 1" <- FALSE ("RL_Read 2")
          }
          frame 6 {
            # "Stand by"
            n94 = local read "Flash"() -> (w512:bool)
            n95 = local write "WDW_Read 1"(w512) -> ()
          }
        }
        n96 = case shown="2" w234 {
          tunnel: [w337 w343 w348 w364 w374 w382 w392 w402 w410 w418 w423] -> w230
          tunnel: w233 -> [_ w343 w353 w364 w374 w382 w392 w402 w410 w418 w423]
          tunnel: w229 -> [_ w346 w356 w361 w370 w381 w391 w401 w409 w415 w422]
          tunnel: [w337 w346 w356 w361 w366 w381 w391 w401 w409 w415 w422] -> w228
          tunnel: [w337 w345 w355 w363 w373 w380 w384 w400 w408 w417 w421] -> w226
          tunnel: w227 -> [_ w345 w355 w363 w373 w380 w388 w400 w408 w417 w421]
          tunnel: [w337 w344 w354 w362 w372 w379 w390 w394 w407 w416 w420] -> w225
          tunnel: w224 -> [_ w344 w354 w362 w372 w379 w390 w398 w407 w416 w420]
          tunnel: w221 -> [_ _ w351 _ w369 _ w387 w397 _ _ _]
          tunnel: w219 -> [_ w341 _ w359 _ w377 _ _ w405 _ _]
          tunnel: w223 -> [_ _ w350 _ w368 _ w386 w396 _ _ _]
          tunnel: w232 -> [_ w342 w349 w360 w367 w378 w385 w395 w406 w414 w419]
          tunnel: [w339 w340 w349 w358 w367 w376 w385 w395 w404 w414 w419] -> w231
          frame 0, Default {
            w337 = T1 {"Stroke Data"=[], "Force Data"=[], "Volt Data 1"=[], "Volt Data 2"=[]} ("Analog Array Out")
            w338 = FALSE ("RL Judge")
            w339 = dbl[] [0.0]  # KnopDistance
            # "WDW L2"
            n97 = shared-variable "My Computer\\AnalogAcquisition.lvlib\\WDW_2_OK"(w338) -> ()  [unwired: 1 in, 1 out]
            "WDW Judge 2" <- w338
          }
          frame 7 {
            # "WDW Distance 1 (Begin Press 0 mm.)"
            n98 = local read "Flash"() -> (w347:bool)
            n99 = Insert Into Array(array=w342, new element=w341) -> (w340:dbl[])  [unwired: 1 in]
            "KnobDistance 2.1" <- w340
            n100 = local write "WDW_Read 2"(w347) -> ()
            n101 = shared-variable "My Computer\\AnalogAcquisition.lvlib\\KnobDistance 2.1"(w340) -> ()  [unwired: 1 in, 1 out]
          }
          frame 1 {
            # "WDW Down Lock"
            n102 = call "WDWAnalog_Recoder.vi"("Lane Number"="Lane 2", "Analog Data In"=w350, "ForceData"=w351, "Analog Array In"=w353) -> ("Analog Array Out"=w348:T1)  [unwired: 7 in]
            "BufferWDWArray 2.1" <- w348
            n103 = local read "Flash"() -> (w357:bool)
            n104 = local write "WDW_Read 2"(w357) -> ()
            n105 = shared-variable "My Computer\\AnalogAcquisition.lvlib\\WDWArray 2.1"(w348) -> ()  [unwired: 1 in, 1 out]
          }
          frame 8 {
            # "Distance 2 (Full Stroke 4.5 mm.)"
            n106 = Insert Into Array(array=w360, new element=w359) -> (w358:dbl[])  [unwired: 1 in]
            "KnobDistance 2.2" <- w358
            n107 = local read "Flash"() -> (w365:bool)
            n108 = local write "WDW_Read 2"(w365) -> ()
            n109 = shared-variable "My Computer\\AnalogAcquisition.lvlib\\KnobDistance 2.2"(w358) -> ()  [unwired: 1 in, 1 out]
          }
          frame 2 {
            # "WDW Down Lock Return"
            n110 = call "WDWAnalog_Recoder.vi"("Lane Number"="Lane 2", "Analog Data In"=w368, "ForceData"=w369, "Analog Array In"=w370) -> ("Analog Array Out"=w366:T1)  [unwired: 7 in]
            "BufferWDWArray 2.2" <- w366
            n111 = local read "Flash"() -> (w375:bool)
            n112 = local write "WDW_Read 2"(w375) -> ()
            n113 = shared-variable "My Computer\\AnalogAcquisition.lvlib\\WDWArray 2.2"(w366) -> ()  [unwired: 1 in, 1 out]
          }
          frame 9 {
            # "Distance 3 (Lock Stroke 3 mm.)"
            n114 = local read "Flash"() -> (w383:bool)
            n115 = Insert Into Array(array=w378, new element=w377) -> (w376:dbl[])  [unwired: 1 in]
            "KnobDistance 2.3" <- w376
            n116 = local write "WDW_Read 2"(w383) -> ()
            n117 = shared-variable "My Computer\\AnalogAcquisition.lvlib\\KnobDistance 2.3"(w376) -> ()  [unwired: 1 in, 1 out]
          }
          frame 3 {
            # "Recode Down Unlock"
            n118 = call "WDWAnalog_Recoder.vi"("Lane Number"="Lane 2", "Analog Data In"=w386, "ForceData"=w387, "Analog Array In"=w388) -> ("Analog Array Out"=w384:T1)  [unwired: 7 in]
            "BufferWDWArray 2.3" <- w384
            n119 = local read "Flash"() -> (w393:bool)
            n120 = local write "WDW_Read 2"(w393) -> ()
            n121 = shared-variable "My Computer\\AnalogAcquisition.lvlib\\WDWArray 2.3"(w384) -> ()  [unwired: 1 in, 1 out]
          }
          frame 4 {
            # "Recode Return Down Unlock"
            n122 = call "WDWAnalog_Recoder.vi"("Lane Number"="Lane 2", "Analog Data In"=w396, "ForceData"=w397, "Analog Array In"=w398) -> ("Analog Array Out"=w394:T1)  [unwired: 7 in]
            "BufferWDWArray 2.4" <- w394
            n123 = local read "Flash"() -> (w403:bool)
            n124 = local write "WDW_Read 2"(w403) -> ()
            n125 = shared-variable "My Computer\\AnalogAcquisition.lvlib\\WDWArray 2.4"(w394) -> ()  [unwired: 1 in, 1 out]
          }
          frame 10 {
            # "Distance 4 (Unpress 0 mm.)"
            n126 = Insert Into Array(array=w406, new element=w405) -> (w404:dbl[])  [unwired: 1 in]
            "KnobDistance 2.4" <- w404
            n127 = local read "Flash"() -> (w411:bool)
            n128 = shared-variable "My Computer\\AnalogAcquisition.lvlib\\KnobDistance 2.4"(w404) -> ()  [unwired: 1 in, 1 out]
            n129 = local write "WDW_Read 2"(w411) -> ()
          }
          frame 5 {
            w412 = TRUE ("RL Judge 2")
            # "Calculate FW & RW Angle"
            n130 = local write "WDW Judge 2"(w412) -> ()
            n131 = shared-variable "My Computer\\AnalogAcquisition.lvlib\\WDW_2_OK"(w412) -> ()  [unwired: 1 in, 1 out]
            "WDW_Read 2" <- FALSE ("RL_Read 2")
          }
          frame 6 {
            # "Stand by"
            n132 = local read "Flash"() -> (w424:bool)
            n133 = local write "WDW_Read 2"(w424) -> ()
          }
        }
        n134 = case shown="0, Default" w292 {
          tunnel: w324 -> [_ w768 w771 w783 w792 w801 w806]
          tunnel: [w759 w763 w771 w783 w792 w801 w806] -> w308
          tunnel: w223 -> [_ w766 w776 w785 w794 _ _]
          tunnel: w323 -> [_ w764 w773 w778 w787 w800 w805]
          tunnel: [w759 w764 w772 w778 w787 w800 w805] -> w307
          tunnel: [w759 w762 w770 w779 w790 w799 w804] -> w270
          tunnel: w269 -> [_ w762 w770 w780 w790 w799 w804]
          tunnel: [w759 w761 w769 w781 w788 w798 w803] -> w268
          tunnel: w267 -> [_ w761 w769 w781 w789 w798 w803]
          frame 0, Default {
            w758 = FALSE ("RL Judge")
            w759 = T2 {"Angle Data"=[], "Force Data"=[], "Volt Data 1"=[], "Volt Data 2"=[]} ("Analog Array Out")
            n135 = shared-variable "My Computer\\AnalogAcquisition.lvlib\\RL_1_OK"(w758) -> ()  [unwired: 1 in, 1 out]
            "RL Judge" <- w758
          }
          frame 1 {
            # "RL Up"
            n136 = call "Analog_Recoder.vi"("Test Name"="RL", "Lane Number"="Lane 1", "Analog Data In"=w766, "Analog Array In"=w768) -> ("Analog Array Out"=w763:T2)  [unwired: 7 in]
            "BufferRLArray 1.1" <- w763
            n137 = local read "Flash"() -> (w760:bool)
            n138 = shared-variable "My Computer\\AnalogAcquisition.lvlib\\RLArray 1.1"(w763) -> ()  [unwired: 1 in, 1 out]
            n139 = local write "RL_Read 1"(w760) -> ()
          }
          frame 2 {
            # "RL Up Return"
            n140 = local read "Flash"() -> (w774:bool)
            n141 = call "Analog_Recoder.vi"("Test Name"="RL", "Lane Number"="Lane 1", "Analog Data In"=w776, "Analog Array In"=w773) -> ("Analog Array Out"=w772:T2)  [unwired: 7 in]
            "BufferRLArray 1.2" <- w772
            n142 = local write "RL_Read 1"(w774) -> ()
            n143 = shared-variable "My Computer\\AnalogAcquisition.lvlib\\RLArray 1.2"(w772) -> ()  [unwired: 1 in, 1 out]
          }
          frame 3 {
            # "RL Down"
            n144 = local read "Flash"() -> (w782:bool)
            n145 = call "Analog_Recoder.vi"("Test Name"="RL", "Lane Number"="Lane 1", "Analog Data In"=w785, "Analog Array In"=w780) -> ("Analog Array Out"=w779:T2)  [unwired: 7 in]
            "BufferRLArray 1.3" <- w779
            n146 = local write "RL_Read 1"(w782) -> ()
            n147 = shared-variable "My Computer\\AnalogAcquisition.lvlib\\RLArray 1.3"(w779) -> ()  [unwired: 1 in, 1 out]
          }
          frame 4 {
            # "RL Down Return"
            n148 = local read "Flash"() -> (w791:bool)
            n149 = call "Analog_Recoder.vi"("Test Name"="RL", "Lane Number"="Lane 1", "Analog Data In"=w794, "Analog Array In"=w789) -> ("Analog Array Out"=w788:T2)  [unwired: 7 in]
            "BufferRLArray 1.4" <- w788
            n150 = local write "RL_Read 1"(w791) -> ()
            n151 = shared-variable "My Computer\\AnalogAcquisition.lvlib\\RLArray 1.4"(w788) -> ()  [unwired: 1 in, 1 out]
          }
          frame 5 {
            w797 = TRUE ("RL Judge")
            # "Calculate FW & RW Angle"
            n152 = local write "RL Judge"(w797) -> ()
            n153 = shared-variable "My Computer\\AnalogAcquisition.lvlib\\RL_1_OK"(w797) -> ()  [unwired: 1 in, 1 out]
            "RL_Read 1" <- FALSE ("RL_Read 1")
          }
          frame 6 {
            # "Stand by"
            n154 = local read "Flash"() -> (w802:bool)
            n155 = local write "RL_Read 1"(w802) -> ()
          }
        }
        n156 = case shown="6" w291 {
          tunnel: w314 -> [_ w717 w728 w732 w741 w752 w757]
          tunnel: [w710 w717 w728 w731 w741 w752 w757] -> w306
          tunnel: w223 -> [_ w712 w722 w729 w745 _ _]
          tunnel: w315 -> [_ w719 w721 w737 w739 w751 w756]
          tunnel: [w710 w719 w721 w737 w738 w751 w756] -> w305
          tunnel: [w710 w713 w726 w730 w742 w750 w755] -> w266
          tunnel: w265 -> [_ w714 w726 w730 w742 w750 w755]
          tunnel: [w710 w718 w720 w735 w740 w749 w754] -> w264
          tunnel: w263 -> [_ w718 w723 w735 w740 w749 w754]
          frame 0, Default {
            w709 = FALSE ("DL Judge")
            w710 = T2 {"Angle Data"=[], "Force Data"=[], "Volt Data 1"=[], "Volt Data 2"=[]} ("Analog Array Out")
            n157 = shared-variable "My Computer\\AnalogAcquisition.lvlib\\DL_2_OK"(w709) -> ()  [unwired: 1 in, 1 out]
            "DoorLock Judge 2" <- w709
          }
          frame 1 {
            # "Door Unlock"
            n158 = call "Analog_Recoder.vi"("Test Name"="DL", "Lane Number"="Lane 2", "Analog Data In"=w712, "Analog Array In"=w714) -> ("Analog Array Out"=w713:T2)  [unwired: 7 in]
            "BufferDLArray 2.3" <- w713
            n159 = local read "Flash"() -> (w711:bool)
            n160 = local write "DL_Read 2"(w711) -> ()
            n161 = shared-variable "My Computer\\AnalogAcquisition.lvlib\\DLArray 2.3"(w713) -> ()  [unwired: 1 in, 1 out]
          }
          frame 2 {
            # "Door Unlock"
            n162 = local read "Flash"() -> (w727:bool)
            n163 = call "Analog_Recoder.vi"("Test Name"="DL", "Lane Number"="Lane 2", "Analog Data In"=w722, "Analog Array In"=w723) -> ("Analog Array Out"=w720:T2)  [unwired: 7 in]
            "BufferDLArray 2.4" <- w720
            n164 = local write "DL_Read 2"(w727) -> ()
            n165 = shared-variable "My Computer\\AnalogAcquisition.lvlib\\DLArray 2.4"(w720) -> ()  [unwired: 1 in, 1 out]
          }
          frame 3 {
            # "Door Lock"
            n166 = local read "Flash"() -> (w736:bool)
            n167 = local write "DL_Read 2"(w736) -> ()
            n168 = call "Analog_Recoder.vi"("Test Name"="DL", "Lane Number"="Lane 2", "Analog Data In"=w729, "Analog Array In"=w732) -> ("Analog Array Out"=w731:T2)  [unwired: 7 in]
            "BufferDLArray 2.1" <- w731
            n169 = shared-variable "My Computer\\AnalogAcquisition.lvlib\\DLArray 2.1"(w731) -> ()  [unwired: 1 in, 1 out]
          }
          frame 4 {
            # "Door Lock Return"
            n170 = local read "Flash"() -> (w743:bool)
            n171 = call "Analog_Recoder.vi"("Test Name"="DL", "Lane Number"="Lane 2", "Analog Data In"=w745, "Analog Array In"=w739) -> ("Analog Array Out"=w738:T2)  [unwired: 7 in]
            "BufferDLArray 2.2" <- w738
            n172 = local write "DL_Read 2"(w743) -> ()
            n173 = shared-variable "My Computer\\AnalogAcquisition.lvlib\\DLArray 2.2"(w738) -> ()  [unwired: 1 in, 1 out]
          }
          frame 5 {
            w748 = TRUE ("DoorLock Judge 2")
            # "Calculate FW & RW Angle"
            n174 = local write "DoorLock Judge 2"(w748) -> ()
            n175 = shared-variable "My Computer\\AnalogAcquisition.lvlib\\DL_2_OK"(w748) -> ()  [unwired: 1 in, 1 out]
            "DL_Read 2" <- FALSE ("DL_Read 2")
          }
          frame 6 {
            # "Stand by"
            n176 = local read "Flash"() -> (w753:bool)
            n177 = local write "DL_Read 2"(w753) -> ()
          }
        }
        n178 = case shown="6" w290 {
          tunnel: w313 -> [_ w670 w671 w685 w694 w703 w708]
          tunnel: [w661 w666 w671 w685 w694 w703 w708] -> w304
          tunnel: w223 -> [_ w668 w678 w687 w696 _ _]
          tunnel: w316 -> [_ w665 w673 w680 w691 w702 w707]
          tunnel: [w661 w665 w672 w680 w691 w702 w707] -> w303
          tunnel: [w661 w664 w675 w682 w692 w701 w706] -> w261
          tunnel: w262 -> [_ w664 w675 w683 w692 w701 w706]
          tunnel: [w661 w663 w674 w681 w689 w700 w705] -> w260
          tunnel: w259 -> [_ w663 w674 w681 w690 w700 w705]
          frame 0, Default {
            w660 = FALSE ("FR Judge")
            w661 = T2 {"Angle Data"=[], "Force Data"=[], "Volt Data 1"=[], "Volt Data 2"=[]} ("Analog Array Out")
            n179 = shared-variable "My Computer\\AnalogAcquisition.lvlib\\FR_2_OK"(w660) -> ()  [unwired: 1 in, 1 out]
            "FR Judge 2" <- w660
          }
          frame 1 {
            # "FR Up"
            n180 = call "Analog_Recoder.vi"("Test Name"="FR", "Lane Number"="Lane 2", "Analog Data In"=w668, "Analog Array In"=w670) -> ("Analog Array Out"=w666:T2)  [unwired: 7 in]
            "BufferFRArray 2.1" <- w666
            n181 = local read "Flash"() -> (w662:bool)
            n182 = shared-variable "My Computer\\AnalogAcquisition.lvlib\\FRArray 2.1"(w666) -> ()  [unwired: 1 in, 1 out]
            n183 = local write "FR_Read 2"(w662) -> ()
          }
          frame 2 {
            # "FR Up Return"
            n184 = call "Analog_Recoder.vi"("Test Name"="FR", "Lane Number"="Lane 2", "Analog Data In"=w678, "Analog Array In"=w673) -> ("Analog Array Out"=w672:T2)  [unwired: 7 in]
            "BufferFRArray 2.2" <- w672
            n185 = local read "Flash"() -> (w676:bool)
            n186 = local write "FR_Read 2"(w676) -> ()
            n187 = shared-variable "My Computer\\AnalogAcquisition.lvlib\\FRArray 2.2"(w672) -> ()  [unwired: 1 in, 1 out]
          }
          frame 3 {
            # "FR Down"
            n188 = local read "Flash"() -> (w684:bool)
            n189 = call "Analog_Recoder.vi"("Test Name"="FR", "Lane Number"="Lane 2", "Analog Data In"=w687, "Analog Array In"=w683) -> ("Analog Array Out"=w682:T2)  [unwired: 7 in]
            "BufferFRArray 2.3" <- w682
            n190 = local write "FR_Read 2"(w684) -> ()
            n191 = shared-variable "My Computer\\AnalogAcquisition.lvlib\\FRArray 2.3"(w682) -> ()  [unwired: 1 in, 1 out]
          }
          frame 4 {
            # "FR Down Return"
            n192 = local read "Flash"() -> (w693:bool)
            n193 = call "Analog_Recoder.vi"("Test Name"="FR", "Lane Number"="Lane 2", "Analog Data In"=w696, "Analog Array In"=w690) -> ("Analog Array Out"=w689:T2)  [unwired: 7 in]
            "BufferFRArray 2.4" <- w689
            n194 = local write "FR_Read 2"(w693) -> ()
            n195 = shared-variable "My Computer\\AnalogAcquisition.lvlib\\FRArray 2.4"(w689) -> ()  [unwired: 1 in, 1 out]
          }
          frame 5 {
            w699 = TRUE ("FR Judge 2")
            # "Calculate FW & RW Angle"
            n196 = local write "FR Judge 2"(w699) -> ()
            n197 = shared-variable "My Computer\\AnalogAcquisition.lvlib\\FR_2_OK"(w699) -> ()  [unwired: 1 in, 1 out]
            "FR_Read 2" <- FALSE ("FR_Read 2")
          }
          frame 6 {
            # "Stand by"
            n198 = local read "Flash"() -> (w704:bool)
            n199 = local write "FR_Read 2"(w704) -> ()
          }
        }
        n200 = case shown="6" w289 {
          tunnel: w317 -> [_ w621 w624 w636 w645 w654 w659]
          tunnel: [w612 w617 w624 w636 w645 w654 w659] -> w302
          tunnel: w223 -> [_ w619 w629 w638 w647 _ _]
          tunnel: w318 -> [_ w616 w623 w631 w640 w653 w658]
          tunnel: [w612 w616 w622 w631 w640 w653 w658] -> w301
          tunnel: [w612 w615 w626 w632 w643 w652 w657] -> w258
          tunnel: w257 -> [_ w615 w626 w633 w643 w652 w657]
          tunnel: [w612 w614 w625 w634 w641 w651 w656] -> w256
          tunnel: w255 -> [_ w614 w625 w634 w642 w651 w656]
          frame 0, Default {
            w611 = FALSE ("RR Judge")
            w612 = T2 {"Angle Data"=[], "Force Data"=[], "Volt Data 1"=[], "Volt Data 2"=[]} ("Analog Array Out")
            n201 = shared-variable "My Computer\\AnalogAcquisition.lvlib\\RR_2_OK"(w611) -> ()  [unwired: 1 in, 1 out]
            "RR Judge 2" <- w611
          }
          frame 1 {
            # "RR Up"
            n202 = call "Analog_Recoder.vi"("Test Name"="RR", "Lane Number"="Lane 2", "Analog Data In"=w619, "Analog Array In"=w621) -> ("Analog Array Out"=w617:T2)  [unwired: 7 in]
            "BufferRRArray 2.1" <- w617
            n203 = local read "Flash"() -> (w613:bool)
            n204 = shared-variable "My Computer\\AnalogAcquisition.lvlib\\RRArray 2.1"(w617) -> ()  [unwired: 1 in, 1 out]
            n205 = local write "RR_Read 2"(w613) -> ()
          }
          frame 2 {
            # "RR Up Return"
            n206 = call "Analog_Recoder.vi"("Test Name"="RR", "Lane Number"="Lane 2", "Analog Data In"=w629, "Analog Array In"=w623) -> ("Analog Array Out"=w622:T2)  [unwired: 7 in]
            "BufferRRArray 2.2" <- w622
            n207 = local read "Flash"() -> (w627:bool)
            n208 = shared-variable "My Computer\\AnalogAcquisition.lvlib\\RRArray 2.2"(w622) -> ()  [unwired: 1 in, 1 out]
            n209 = local write "RR_Read 2"(w627) -> ()
          }
          frame 3 {
            # "RR Down"
            n210 = local read "Flash"() -> (w635:bool)
            n211 = call "Analog_Recoder.vi"("Test Name"="RR", "Lane Number"="Lane 2", "Analog Data In"=w638, "Analog Array In"=w633) -> ("Analog Array Out"=w632:T2)  [unwired: 7 in]
            "BufferRRArray 2.3" <- w632
            n212 = local write "RR_Read 2"(w635) -> ()
            n213 = shared-variable "My Computer\\AnalogAcquisition.lvlib\\RRArray 2.3"(w632) -> ()  [unwired: 1 in, 1 out]
          }
          frame 4 {
            # "RR Down Return"
            n214 = local read "Flash"() -> (w644:bool)
            n215 = call "Analog_Recoder.vi"("Test Name"="RR", "Lane Number"="Lane 2", "Analog Data In"=w647, "Analog Array In"=w642) -> ("Analog Array Out"=w641:T2)  [unwired: 7 in]
            "BufferRRArray 2.4" <- w641
            n216 = local write "RR_Read 2"(w644) -> ()
            n217 = shared-variable "My Computer\\AnalogAcquisition.lvlib\\RRArray 2.4"(w641) -> ()  [unwired: 1 in, 1 out]
          }
          frame 5 {
            w650 = TRUE ("RR Judge 2")
            # "Calculate FW & RW Angle"
            n218 = local write "RR Judge 2"(w650) -> ()
            n219 = shared-variable "My Computer\\AnalogAcquisition.lvlib\\RR_2_OK"(w650) -> ()  [unwired: 1 in, 1 out]
            "RR_Read 2" <- FALSE ("RR_Read 2")
          }
          frame 6 {
            # "Stand by"
            n220 = local read "Flash"() -> (w655:bool)
            n221 = local write "RR_Read 2"(w655) -> ()
          }
        }
        n222 = case shown="1" w288 {
          tunnel: w320 -> [_ w572 w575 w587 w596 w605 w610]
          tunnel: [w563 w568 w575 w587 w596 w605 w610] -> w300
          tunnel: w223 -> [_ w570 w580 w589 w598 _ _]
          tunnel: w319 -> [_ w567 w577 w582 w591 w604 w609]
          tunnel: [w563 w567 w576 w582 w591 w604 w609] -> w299
          tunnel: [w563 w566 w574 w583 w594 w603 w608] -> w254
          tunnel: w253 -> [_ w566 w574 w584 w594 w603 w608]
          tunnel: [w563 w565 w573 w585 w592 w602 w607] -> w252
          tunnel: w251 -> [_ w565 w573 w585 w593 w602 w607]
          frame 0, Default {
            w562 = FALSE ("FL Judge")
            w563 = T2 {"Angle Data"=[], "Force Data"=[], "Volt Data 1"=[], "Volt Data 2"=[]} ("Analog Array Out")
            n223 = shared-variable "My Computer\\AnalogAcquisition.lvlib\\FL_2_OK"(w562) -> ()  [unwired: 1 in, 1 out]
            "FL Judge 2" <- w562
          }
          frame 1 {
            # "FL Up"
            n224 = call "Analog_Recoder.vi"("Test Name"="FL", "Lane Number"="Lane 2", "Analog Data In"=w570, "Analog Array In"=w572) -> ("Analog Array Out"=w568:T2)  [unwired: 7 in]
            "BufferFLArray 2.1" <- w568
            n225 = local read "Flash"() -> (w564:bool)
            n226 = shared-variable "My Computer\\AnalogAcquisition.lvlib\\FLArray 2.1"(w568) -> ()  [unwired: 1 in, 1 out]
            n227 = local write "FL_Read 2"(w564) -> ()
          }
          frame 2 {
            # "FL Up"
            n228 = call "Analog_Recoder.vi"("Test Name"="FL", "Lane Number"="Lane 2", "Analog Data In"=w580, "Analog Array In"=w577) -> ("Analog Array Out"=w576:T2)  [unwired: 7 in]
            "BufferFLArray 2.2" <- w576
            n229 = local read "Flash"() -> (w578:bool)
            n230 = shared-variable "My Computer\\AnalogAcquisition.lvlib\\FLArray 2.2"(w576) -> ()  [unwired: 1 in, 1 out]
            n231 = local write "FL_Read 2"(w578) -> ()
          }
          frame 3 {
            # "FL Down"
            n232 = local read "Flash"() -> (w586:bool)
            n233 = call "Analog_Recoder.vi"("Test Name"="FL", "Lane Number"="Lane 2", "Analog Data In"=w589, "Analog Array In"=w584) -> ("Analog Array Out"=w583:T2)  [unwired: 7 in]
            "BufferFLArray 2.3" <- w583
            n234 = local write "FL_Read 2"(w586) -> ()
            n235 = shared-variable "My Computer\\AnalogAcquisition.lvlib\\FLArray 2.3"(w583) -> ()  [unwired: 1 in, 1 out]
          }
          frame 4 {
            # "FL Down Return"
            n236 = local read "Flash"() -> (w595:bool)
            n237 = call "Analog_Recoder.vi"("Test Name"="FL", "Lane Number"="Lane 2", "Analog Data In"=w598, "Analog Array In"=w593) -> ("Analog Array Out"=w592:T2)  [unwired: 7 in]
            "BufferFLArray 2.4" <- w592
            n238 = local write "FL_Read 2"(w595) -> ()
            n239 = shared-variable "My Computer\\AnalogAcquisition.lvlib\\FLArray 2.4"(w592) -> ()  [unwired: 1 in, 1 out]
          }
          frame 5 {
            w601 = TRUE ("FL Judge 2")
            # "Calculate FW & RW Angle"
            n240 = local write "FL Judge 2"(w601) -> ()
            n241 = shared-variable "My Computer\\AnalogAcquisition.lvlib\\FL_2_OK"(w601) -> ()  [unwired: 1 in, 1 out]
            "FL_Read 2" <- FALSE ("FL_Read 2")
          }
          frame 6 {
            # "Stand by"
            n242 = local read "Flash"() -> (w606:bool)
            n243 = local write "FL_Read 2"(w606) -> ()
          }
        }
        n244 = case shown="1" w287 {
          tunnel: w321 -> [_ w523 w526 w538 w547 w556 w561]
          tunnel: [w514 w519 w526 w538 w547 w556 w561] -> w298
          tunnel: w223 -> [_ w521 w531 w540 w549 _ _]
          tunnel: w322 -> [_ w518 w525 w533 w542 w555 w560]
          tunnel: [w514 w518 w524 w533 w542 w555 w560] -> w297
          tunnel: w250 -> [_ w517 w528 w535 w545 w554 w559]
          tunnel: w249 -> [_ w516 w527 w536 w544 w553 w558]
          tunnel: [w514 w517 w528 w534 w545 w554 w559] -> w248
          tunnel: [w514 w516 w527 w536 w543 w553 w558] -> w247
          frame 0, Default {
            w513 = FALSE ("RL Judge")
            w514 = T2 {"Angle Data"=[], "Force Data"=[], "Volt Data 1"=[], "Volt Data 2"=[]} ("Analog Array Out")
            n245 = shared-variable "My Computer\\AnalogAcquisition.lvlib\\RL_2_OK"(w513) -> ()  [unwired: 1 in, 1 out]
            "RL Judge 2" <- w513
          }
          frame 1 {
            # "RL Up"
            n246 = call "Analog_Recoder.vi"("Test Name"="RL", "Lane Number"="Lane 2", "Analog Data In"=w521, "Analog Array In"=w523) -> ("Analog Array Out"=w519:T2)  [unwired: 7 in]
            "BufferRLArray 2.1" <- w519
            n247 = local read "Flash"() -> (w515:bool)
            n248 = shared-variable "My Computer\\AnalogAcquisition.lvlib\\RLArray 2.1"(w519) -> ()  [unwired: 1 in, 1 out]
            n249 = local write "RL_Read 2"(w515) -> ()
          }
          frame 2 {
            # "RL Up Return"
            n250 = call "Analog_Recoder.vi"("Test Name"="RL", "Lane Number"="Lane 2", "Analog Data In"=w531, "Analog Array In"=w525) -> ("Analog Array Out"=w524:T2)  [unwired: 7 in]
            "BufferRLArray 2.2" <- w524
            n251 = local read "Flash"() -> (w529:bool)
            n252 = shared-variable "My Computer\\AnalogAcquisition.lvlib\\RLArray 2.2"(w524) -> ()  [unwired: 1 in, 1 out]
            n253 = local write "RL_Read 2"(w529) -> ()
          }
          frame 3 {
            # "RL Down"
            n254 = local read "Flash"() -> (w537:bool)
            n255 = call "Analog_Recoder.vi"("Test Name"="RL", "Lane Number"="Lane 2", "Analog Data In"=w540, "Analog Array In"=w535) -> ("Analog Array Out"=w534:T2)  [unwired: 7 in]
            "BufferRLArray 2.3" <- w534
            n256 = local write "RL_Read 2"(w537) -> ()
            n257 = shared-variable "My Computer\\AnalogAcquisition.lvlib\\RLArray 2.3"(w534) -> ()  [unwired: 1 in, 1 out]
          }
          frame 4 {
            # "RL Down Return"
            n258 = local read "Flash"() -> (w546:bool)
            n259 = call "Analog_Recoder.vi"("Test Name"="RL", "Lane Number"="Lane 2", "Analog Data In"=w549, "Analog Array In"=w544) -> ("Analog Array Out"=w543:T2)  [unwired: 7 in]
            "BufferRLArray 2.4" <- w543
            n260 = local write "RL_Read 2"(w546) -> ()
            n261 = shared-variable "My Computer\\AnalogAcquisition.lvlib\\RLArray 2.4"(w543) -> ()  [unwired: 1 in, 1 out]
          }
          frame 5 {
            w552 = TRUE ("RL Judge 2")
            # "Calculate FW & RW Angle"
            n262 = local write "RL Judge 2"(w552) -> ()
            n263 = shared-variable "My Computer\\AnalogAcquisition.lvlib\\RL_2_OK"(w552) -> ()  [unwired: 1 in, 1 out]
            "RL_Read 2" <- FALSE ("RL_Read 2")
          }
          frame 6 {
            # "Stand by"
            n264 = local read "Flash"() -> (w557:bool)
            n265 = local write "RL_Read 2"(w557) -> ()
          }
        }
        n266 = case shown="0, Default" w296 {
          tunnel: w336 -> [_ w963 w972 w982 w986 w997 w1002]
          tunnel: [w955 w963 w972 w977 w986 w997 w1002] -> w334
          tunnel: w223 -> [_ w960 w971 w980 w990 _ _]
          tunnel: w335 -> [_ w958 w966 w979 w985 w996 w1001]
          tunnel: [w955 w958 w966 w979 w984 w996 w1001] -> w333
          tunnel: [w955 w956 w969 w976 w988 w995 w1000] -> w285
          tunnel: w286 -> [_ w959 w969 w976 w988 w995 w1000]
          tunnel: [w955 w961 w967 w975 w987 w994 w999] -> w284
          tunnel: w283 -> [_ w961 w968 w975 w987 w994 w999]
          frame 0, Default {
            w954 = FALSE ("DL Judge")
            w955 = T2 {"Angle Data"=[], "Force Data"=[], "Volt Data 1"=[], "Volt Data 2"=[]} ("Analog Array Out")
            n267 = shared-variable "My Computer\\AnalogAcquisition.lvlib\\DL_1_OK"(w954) -> ()  [unwired: 1 in, 1 out]
            "DoorLock Judge" <- w954
          }
          frame 1 {
            # "Door Unlock"
            n268 = call "Analog_Recoder.vi"("Test Name"="DL", "Lane Number"="Lane 1", "Analog Data In"=w960, "Analog Array In"=w959) -> ("Analog Array Out"=w956:T2)  [unwired: 7 in]
            "BufferDLArray 1.3" <- w956
            n269 = local read "Flash"() -> (w957:bool)
            n270 = local write "DL_Read 1"(w957) -> ()
            n271 = shared-variable "My Computer\\AnalogAcquisition.lvlib\\DLArray 1.3"(w956) -> ()  [unwired: 1 in, 1 out]
          }
          frame 2 {
            # "Door Unlock Return"
            n272 = local read "Flash"() -> (w965:bool)
            n273 = call "Analog_Recoder.vi"("Test Name"="DL", "Lane Number"="Lane 1", "Analog Data In"=w971, "Analog Array In"=w968) -> ("Analog Array Out"=w967:T2)  [unwired: 7 in]
            "BufferDLArray 1.4" <- w967
            n274 = local write "DL_Read 1"(w965) -> ()
            n275 = shared-variable "My Computer\\AnalogAcquisition.lvlib\\DLArray 1.4"(w967) -> ()  [unwired: 1 in, 1 out]
          }
          frame 3 {
            # "Door Lock"
            n276 = local read "Flash"() -> (w974:bool)
            n277 = call "Analog_Recoder.vi"("Test Name"="DL", "Lane Number"="Lane 1", "Analog Data In"=w980, "Analog Array In"=w982) -> ("Analog Array Out"=w977:T2)  [unwired: 7 in]
            "BufferDLArray 1.1" <- w977
            n278 = local write "DL_Read 1"(w974) -> ()
            n279 = shared-variable "My Computer\\AnalogAcquisition.lvlib\\DLArray 1.1"(w977) -> ()  [unwired: 1 in, 1 out]
          }
          frame 4 {
            # "Door Lock Return"
            n280 = local read "Flash"() -> (w983:bool)
            n281 = call "Analog_Recoder.vi"("Test Name"="DL", "Lane Number"="Lane 1", "Analog Data In"=w990, "Analog Array In"=w985) -> ("Analog Array Out"=w984:T2)  [unwired: 7 in]
            "BufferDLArray 1.2" <- w984
            n282 = local write "DL_Read 1"(w983) -> ()
            n283 = shared-variable "My Computer\\AnalogAcquisition.lvlib\\DLArray 1.2"(w984) -> ()  [unwired: 1 in, 1 out]
          }
          frame 5 {
            w993 = TRUE ("DoorLock Judge")
            # "Calculate FW & RW Angle"
            n284 = local write "DoorLock Judge"(w993) -> ()
            n285 = shared-variable "My Computer\\AnalogAcquisition.lvlib\\DL_1_OK"(w993) -> ()  [unwired: 1 in, 1 out]
            "DL_Read 1" <- FALSE ("DL_Read 1")
          }
          frame 6 {
            # "Stand by"
            n286 = local read "Flash"() -> (w998:bool)
            n287 = local write "DL_Read 1"(w998) -> ()
          }
        }
        n288 = case shown="5" w295 {
          tunnel: w332 -> [_ w909 w916 w927 w941 w948 w951]
          tunnel: [w906 w909 w916 w926 w941 w948 w951] -> w330
          tunnel: w223 -> [_ w914 w923 w932 w939 _ _]
          tunnel: w331 -> [_ w913 w922 w925 w940 w947 w950]
          tunnel: [w906 w913 w922 w925 w936 w947 w950] -> w329
          tunnel: [w906 w908 w919 w928 w935 w946 w953] -> w282
          tunnel: w281 -> [_ w910 w919 w928 w935 w946 w953]
          tunnel: [w906 w911 w917 w929 w934 w945 w952] -> w280
          tunnel: w279 -> [_ w911 w918 w929 w934 w945 w952]
          frame 0, Default {
            w905 = FALSE ("FR Judge")
            w906 = T2 {"Angle Data"=[], "Force Data"=[], "Volt Data 1"=[], "Volt Data 2"=[]} ("Analog Array Out")
            n289 = shared-variable "My Computer\\AnalogAcquisition.lvlib\\FR_1_OK"(w905) -> ()  [unwired: 1 in, 1 out]
            "FR Judge" <- w905
          }
          frame 1 {
            # "FR Up"
            n290 = call "Analog_Recoder.vi"("Test Name"="FR", "Lane Number"="Lane 1", "Analog Data In"=w914, "Analog Array In"=w910) -> ("Analog Array Out"=w908:T2)  [unwired: 7 in]
            "BufferFRArray 1.1" <- w908
            n291 = local read "Flash"() -> (w907:bool)
            n292 = local write "FR_Read 1"(w907) -> ()
            n293 = shared-variable "My Computer\\AnalogAcquisition.lvlib\\FRArray 1.1"(w908) -> ()  [unwired: 1 in, 1 out]
          }
          frame 2 {
            # "FR Up Return"
            n294 = local read "Flash"() -> (w920:bool)
            n295 = call "Analog_Recoder.vi"("Test Name"="FR", "Lane Number"="Lane 1", "Analog Data In"=w923, "Analog Array In"=w918) -> ("Analog Array Out"=w917:T2)  [unwired: 7 in]
            "BufferFRArray 1.2" <- w917
            n296 = local write "FR_Read 1"(w920) -> ()
            n297 = shared-variable "My Computer\\AnalogAcquisition.lvlib\\FRArray 1.2"(w917) -> ()  [unwired: 1 in, 1 out]
          }
          frame 3 {
            # "FR Down"
            n298 = local read "Flash"() -> (w930:bool)
            n299 = call "Analog_Recoder.vi"("Test Name"="FR", "Lane Number"="Lane 1", "Analog Data In"=w932, "Analog Array In"=w927) -> ("Analog Array Out"=w926:T2)  [unwired: 7 in]
            "BufferFRArray 1.3" <- w926
            n300 = local write "FR_Read 1"(w930) -> ()
            n301 = shared-variable "My Computer\\AnalogAcquisition.lvlib\\FRArray 1.3"(w926) -> ()  [unwired: 1 in, 1 out]
          }
          frame 4 {
            # "FR Down Return"
            n302 = local read "Flash"() -> (w937:bool)
            n303 = call "Analog_Recoder.vi"("Test Name"="FR", "Lane Number"="Lane 1", "Analog Data In"=w939, "Analog Array In"=w940) -> ("Analog Array Out"=w936:T2)  [unwired: 7 in]
            "BufferFRArray 1.4" <- w936
            n304 = local write "FR_Read 1"(w937) -> ()
            n305 = shared-variable "My Computer\\AnalogAcquisition.lvlib\\FRArray 1.4"(w936) -> ()  [unwired: 1 in, 1 out]
          }
          frame 5 {
            w944 = TRUE ("FR Judge")
            # "Calculate FW & RW Angle"
            n306 = local write "FR Judge"(w944) -> ()
            n307 = shared-variable "My Computer\\AnalogAcquisition.lvlib\\FR_1_OK"(w944) -> ()  [unwired: 1 in, 1 out]
            "FR_Read 1" <- FALSE ("FR_Read 1")
          }
          frame 6 {
            # "Stand by"
            n308 = local read "Flash"() -> (w949:bool)
            n309 = local write "FR_Read 1"(w949) -> ()
          }
        }
        n310 = case shown="6" w294 {
          tunnel: w328 -> [_ w866 w871 w881 w890 w899 w904]
          tunnel: [w857 w861 w871 w881 w890 w899 w904] -> w312
          tunnel: w223 -> [_ w864 w874 w883 w892 _ _]
          tunnel: w327 -> [_ w862 w868 w878 w885 w898 w903]
          tunnel: [w857 w862 w867 w878 w885 w898 w903] -> w311
          tunnel: [w857 w860 w870 w876 w888 w897 w902] -> w278
          tunnel: w277 -> [_ w860 w870 w877 w888 w897 w902]
          tunnel: [w857 w859 w869 w879 w886 w896 w901] -> w276
          tunnel: w275 -> [_ w859 w869 w879 w887 w896 w901]
          frame 0, Default {
            w856 = FALSE ("RR Judge")
            w857 = T2 {"Angle Data"=[], "Force Data"=[], "Volt Data 1"=[], "Volt Data 2"=[]} ("Analog Array Out")
            n311 = shared-variable "My Computer\\AnalogAcquisition.lvlib\\RR_1_OK"(w856) -> ()  [unwired: 1 in, 1 out]
            "RR Judge" <- w856
          }
          frame 1 {
            # "RR Up"
            n312 = call "Analog_Recoder.vi"("Test Name"="RR", "Lane Number"="Lane 1", "Analog Data In"=w864, "Analog Array In"=w866) -> ("Analog Array Out"=w861:T2)  [unwired: 7 in]
            "BufferRRArray 1.1" <- w861
            n313 = local read "Flash"() -> (w858:bool)
            n314 = local write "RR_Read 1"(w858) -> ()
            n315 = shared-variable "My Computer\\AnalogAcquisition.lvlib\\RRArray 1.1"(w861) -> ()  [unwired: 1 in, 1 out]
          }
          frame 2 {
            # "RR Up Return"
            n316 = local read "Flash"() -> (w872:bool)
            n317 = call "Analog_Recoder.vi"("Test Name"="RR", "Lane Number"="Lane 1", "Analog Data In"=w874, "Analog Array In"=w868) -> ("Analog Array Out"=w867:T2)  [unwired: 7 in]
            "BufferRRArray 1.2" <- w867
            n318 = local write "RR_Read 1"(w872) -> ()
            n319 = shared-variable "My Computer\\AnalogAcquisition.lvlib\\RRArray 1.2"(w867) -> ()  [unwired: 1 in, 1 out]
          }
          frame 3 {
            # "RR Down"
            n320 = local read "Flash"() -> (w880:bool)
            n321 = call "Analog_Recoder.vi"("Test Name"="RR", "Lane Number"="Lane 1", "Analog Data In"=w883, "Analog Array In"=w877) -> ("Analog Array Out"=w876:T2)  [unwired: 7 in]
            "BufferRRArray 1.3" <- w876
            n322 = local write "RR_Read 1"(w880) -> ()
            n323 = shared-variable "My Computer\\AnalogAcquisition.lvlib\\RRArray 1.3"(w876) -> ()  [unwired: 1 in, 1 out]
          }
          frame 4 {
            # "RR Down"
            n324 = local read "Flash"() -> (w889:bool)
            n325 = call "Analog_Recoder.vi"("Test Name"="RR", "Lane Number"="Lane 1", "Analog Data In"=w892, "Analog Array In"=w887) -> ("Analog Array Out"=w886:T2)  [unwired: 7 in]
            "BufferRRArray 1.4" <- w886
            n326 = local write "RL_Read 1"(w889) -> ()
            n327 = shared-variable "My Computer\\AnalogAcquisition.lvlib\\RRArray 1.4"(w886) -> ()  [unwired: 1 in, 1 out]
          }
          frame 5 {
            w895 = TRUE ("RR Judge")
            # "Calculate FW & RW Angle"
            n328 = local write "RR Judge"(w895) -> ()
            n329 = shared-variable "My Computer\\AnalogAcquisition.lvlib\\RR_1_OK"(w895) -> ()  [unwired: 1 in, 1 out]
            "RR_Read 1" <- FALSE ("RR_Read 1")
          }
          frame 6 {
            # "Stand by"
            n330 = local read "Flash"() -> (w900:bool)
            n331 = local write "RL_Read 1"(w900) -> ()
          }
        }
        n332 = case shown="6" w293 {
          tunnel: w325 -> [_ w817 w820 w832 w841 w850 w855]
          tunnel: [w808 w812 w820 w832 w841 w850 w855] -> w310
          tunnel: w223 -> [_ w815 w825 w834 w843 _ _]
          tunnel: w326 -> [_ w813 w822 w830 w836 w849 w854]
          tunnel: [w808 w813 w821 w830 w836 w849 w854] -> w309
          tunnel: [w808 w811 w819 w829 w839 w848 w853] -> w273
          tunnel: w274 -> [_ w811 w819 w828 w839 w848 w853]
          tunnel: [w808 w810 w818 w827 w837 w847 w852] -> w272
          tunnel: w271 -> [_ w810 w818 w827 w838 w847 w852]
          frame 0, Default {
            w807 = FALSE ("FL Judge")
            w808 = T2 {"Angle Data"=[], "Force Data"=[], "Volt Data 1"=[], "Volt Data 2"=[]} ("Analog Array Out")
            n333 = shared-variable "My Computer\\AnalogAcquisition.lvlib\\FL_1_OK"(w807) -> ()  [unwired: 1 in, 1 out]
            "FL Judge" <- w807
          }
          frame 1 {
            # "FL Up"
            n334 = call "Analog_Recoder.vi"("Test Name"="FL", "Lane Number"="Lane 1", "Analog Data In"=w815, "Analog Array In"=w817) -> ("Analog Array Out"=w812:T2)  [unwired: 7 in]
            "BufferFLArray 1.1" <- w812
            n335 = local read "Flash"() -> (w809:bool)
            n336 = shared-variable "My Computer\\AnalogAcquisition.lvlib\\FLArray 1.1"(w812) -> ()  [unwired: 1 in, 1 out]
            n337 = local write "FL_Read 1"(w809) -> ()
          }
          frame 2 {
            # "FL Up Return"
            n338 = local read "Flash"() -> (w823:bool)
            n339 = call "Analog_Recoder.vi"("Test Name"="FL", "Lane Number"="Lane 1", "Analog Data In"=w825, "Analog Array In"=w822) -> ("Analog Array Out"=w821:T2)  [unwired: 7 in]
            "BufferFLArray 1.2" <- w821
            n340 = local write "FL_Read 1"(w823) -> ()
            n341 = shared-variable "My Computer\\AnalogAcquisition.lvlib\\FLArray 1.2"(w821) -> ()  [unwired: 1 in, 1 out]
          }
          frame 3 {
            # "FL Down"
            n342 = local read "Flash"() -> (w831:bool)
            n343 = call "Analog_Recoder.vi"("Test Name"="FL", "Lane Number"="Lane 1", "Analog Data In"=w834, "Analog Array In"=w828) -> ("Analog Array Out"=w829:T2)  [unwired: 7 in]
            "BufferFLArray 1.3" <- w829
            n344 = local write "FL_Read 1"(w831) -> ()
            n345 = shared-variable "My Computer\\AnalogAcquisition.lvlib\\FLArray 1.3"(w829) -> ()  [unwired: 1 in, 1 out]
          }
          frame 4 {
            # "FL Down Return"
            n346 = local read "Flash"() -> (w840:bool)
            n347 = call "Analog_Recoder.vi"("Test Name"="FL", "Lane Number"="Lane 1", "Analog Data In"=w843, "Analog Array In"=w838) -> ("Analog Array Out"=w837:T2)  [unwired: 7 in]
            "BufferFLArray 1.4" <- w837
            n348 = local write "FL_Read 1"(w840) -> ()
            n349 = shared-variable "My Computer\\AnalogAcquisition.lvlib\\FLArray 1.4"(w837) -> ()  [unwired: 1 in, 1 out]
          }
          frame 5 {
            w846 = TRUE ("FL Judge")
            # "Calculate FW & RW Angle"
            n350 = local write "FL Judge"(w846) -> ()
            n351 = shared-variable "My Computer\\AnalogAcquisition.lvlib\\FL_1_OK"(w846) -> ()  [unwired: 1 in, 1 out]
            "FL_Read 1" <- FALSE ("FL_Read 1")
          }
          frame 6 {
            # "Stand by"
            n352 = local read "Flash"() -> (w851:bool)
            n353 = local write "FL_Read 1"(w851) -> ()
          }
        }
      }
    }
    n354 = shared-variable "My Computer\\AnalogAcquisition.lvlib\\ST_WDW_Read 1"(w44) -> ()  [unwired: 1 in, 1 out]
    n355 = shared-variable "My Computer\\AnalogAcquisition.lvlib\\ST_WDW_Read 2"(w43) -> ()  [unwired: 1 in, 1 out]
    n356 = shared-variable "My Computer\\AnalogAcquisition.lvlib\\ST_DL_Read 1"(w73) -> ()  [unwired: 1 in, 1 out]
    n357 = shared-variable "My Computer\\AnalogAcquisition.lvlib\\ST_RR_Read 1"(w75) -> ()  [unwired: 1 in, 1 out]
    n358 = shared-variable "My Computer\\AnalogAcquisition.lvlib\\ST_DL_Read 2"(w78) -> ()  [unwired: 1 in, 1 out]
    n359 = shared-variable "My Computer\\AnalogAcquisition.lvlib\\ST_RR_Read 2"(w72) -> ()  [unwired: 1 in, 1 out]
    n360 = shared-variable "My Computer\\AnalogAcquisition.lvlib\\ST_FR_Read 1"(w74) -> ()  [unwired: 1 in, 1 out]
    n361 = shared-variable "My Computer\\AnalogAcquisition.lvlib\\ST_RL_Read 1"(w77) -> ()  [unwired: 1 in, 1 out]
    n362 = shared-variable "My Computer\\AnalogAcquisition.lvlib\\ST_FR_Read 2"(w79) -> ()  [unwired: 1 in, 1 out]
    n363 = shared-variable "My Computer\\AnalogAcquisition.lvlib\\ST_RL_Read 2"(w71) -> ()  [unwired: 1 in, 1 out]
    n364 = shared-variable "My Computer\\AnalogAcquisition.lvlib\\ST_FL_Read 1"(w76) -> ()  [unwired: 1 in, 1 out]
    n365 = shared-variable "My Computer\\AnalogAcquisition.lvlib\\ST_FL_Read 2"(w80) -> ()  [unwired: 1 in, 1 out]
    n366 = shared-variable "My Computer\\AnalogAcquisition.lvlib\\Shut Down"() -> (w81:bool)  [unwired: 1 in, 1 out]
    n367 = call "PulseFlash.vi"("Time Target (ms)"=500) -> ("Flash"=→"Flash":bool)  [unwired: 4 in]
    n368 = call "SamplingRate.vi"("Loop In"=w70) -> ("SamplingRate"=→"SamplingRate":i32)  [unwired: 4 in]
    n369 = Or(x="stop", y=w81) -> (x .or. y?=w45:bool)
  }
  n370 = case shown="True" w6 {
    frame False {
    }
    frame True {
      n371 = Quit LabVIEW(quit? (T)=FALSE) -> ()
    }
  }
  n372 = disable-structure shown="Enabled" {
    disable-tunnel: w2 -> [w1011 _]
    disable-tunnel: w1 -> [w1010 _]
    frame Enabled {
      n373 = call <vilib>:"DAQmx Stop Task.vi"("task/channels in"=w1011, "error in"=w1010) -> ("error out"=w1009:errorcluster)  [unwired: 12 in, 1 out]
      n374 = call <vilib>:"Clear Errors.vi"("error in (no error)"=w1009) -> ()  [unwired: 5 in, 2 out]
    }
    frame Disabled {
    }
  }
  n375 = disable-structure shown="Enabled" {
    disable-tunnel: w9 -> [w1014 _]
    disable-tunnel: w8 -> [w1013 _]
    frame Enabled {
      n376 = call <vilib>:"DAQmx Stop Task.vi"("task/channels in"=w1014, "error in"=w1013) -> ("error out"=w1012:errorcluster)  [unwired: 12 in, 1 out]
      n377 = call <vilib>:"Clear Errors.vi"("error in (no error)"=w1012) -> ()  [unwired: 5 in, 2 out]
    }
    frame Disabled {
    }
  }
  n378 = disable-structure shown="Disabled" {
    frame Disabled {
    }
    frame Enabled {
    }
  }
  n379 = disable-structure shown="Disabled" {
    frame Disabled {
      n380 = local read item#-1() -> ()  [unwired: 1 out]
      n381 = local read item#-1() -> ()  [unwired: 1 out]
      n382 = local read item#-1() -> ()  [unwired: 1 out]
      n383 = local read item#-1() -> ()  [unwired: 1 out]
      n384 = local read item#-1() -> ()  [unwired: 1 out]
      n385 = local read item#-1() -> ()  [unwired: 1 out]
      n386 = local read item#-1() -> ()  [unwired: 1 out]
      n387 = local read item#-1() -> ()  [unwired: 1 out]
      n388 = local read item#-1() -> ()  [unwired: 1 out]
      n389 = local read item#-1() -> ()  [unwired: 1 out]
      n390 = local read item#-1() -> ()  [unwired: 1 out]
      n391 = local read item#-1() -> ()  [unwired: 1 out]
      n392 = local read item#-1() -> ()  [unwired: 1 out]
      n393 = local read item#-1() -> ()  [unwired: 1 out]
    }
    frame Enabled {
    }
  }
